vi "RANGE Gas Meters.vi"() -> ()   [LabVIEW 2023]
uses:
  Type Definitions/RANGE DAQ Data Four Meters.ctl
  Type Definitions/RANGE DAQ Data.ctl
  Drivers/Omega FMA-1600A Series Gas Flow Meter/Type Definitions/FMA1600A Gas Type.ctl
  Drivers/Omega FMA-1600A Series Gas Flow Meter/Type Definitions/FMA1600A Units String.ctl
  Drivers/Alicat Gas Meter Driver/Sub-VIs/Units of Measure.ctl
  Drivers/Alicat Gas Meter Driver/Sub-VIs/Data Frame.ctl
  Type Definitions/RANGE GAS Data.ctl
  Type Definitions/RANGE Panel Data.ctl
  Type Definitions/RANGE ANSI Rate.ctl
  Type Definitions/RANGE Meter Selector 1-2.ctl
  Type Definitions/RANGE Meter Selector 3-4.ctl
  Type Definitions/RANGE Meter Selector 5-6.ctl
  Type Definitions/RANGE Tab Control 2.ctl
  Drivers/Omega FMA-1600A Series Gas Flow Meter/Type Definitions/FMA1600A Commands.ctl
  ValveTester/LabVIEW/Controls/GLVT-Stepper-EnableState.ctl
  ValveTester/LabVIEW/Controls/GLVT-FlowmeterBankSelection.ctl
  ValveTester/LabVIEW/Controls/GLVT-Stepper-RotateDirection.ctl
  Drivers/Inficon Fusion Micro GC/Type Definitions/Inficon IP Address.ctl
  <vilib>/NI/Modbus Library/API/Master/Modbus Master.lvclass
  Utility/Type Definitions/UTILITY Notifier.ctl
  ValveTester/LabVIEW/Controls/GLVT-States.ctl
  Utility/Custom Pallet Controls/Custom Pallet DBL.ctl
  ValveTester/LabVIEW/Controls/GLVT-FGV-States.ctl
  Type Definitions/Range Meter Bank.ctl
  <vilib>/Analysis/baseanly.llb/Mean (DBL).vi
  <vilib>/Analysis/NI_AALBase.lvlib
panel:
  out "GLVT-Filename DTS":string caption="Filename DTS"
  out "GLVT-End Data Collection":bool caption="End Data Collection"
  out "GLVT-Current Angle Array Location":i32 caption="Current Angle Array Location"
  out "GLVT-Row Length":i32
  out "GLVT-Rotate Direction":T1 caption="Rotate Direction"
  in  "Tab Control 2":T2
  out "Bank 3 Gas Pres 2":string
  out "Bank 3 Gas Temp 2":string
  out "Bank 3 Tot. Flow 2":string
  out "Bank 3 Vol Flow 2":string
  out "Bank 3 Mass Flow 2":string
  out "Bank 2 Gas Pres":string
  out "Bank 2 Gas Temp":string
  out "Bank 2 Tot. Flow":string
  out "Bank 2 Vol Flow":string
  out "Bank 2 Mass Flow":string
  out "Bank 1 Gas Pres 2":string
  out "Bank 1 Gas Temp 2":string
  out "Bank 1 Tot. Flow 2":string
  out "Bank 1 Vol Flow 2":string
  in  "Tare Meter Bank 3":bool
  in  "Reset Totalizer Bank 3":bool
  in  "Change Gas Meter Bank 3":bool
  in  "Gas Type 3":T3
  in  "Tare Meter Bank 2":bool
  in  "Reset Totalizer Bank 2":bool
  in  "Change Gas Meter Bank 2":bool
  in  "Gas Type 2":T3
  in  "Tare Meter Bank 1":bool
  in  "Reset Totalizer Bank 1":bool
  out "Flow Rate":dbl caption="Flow Rate (BTU/hr)" format="%#_5f"
  out "DisplayChart":cluster{"Flow Rate (BTU/HR)":dbl}(graph)
  in  "HeatingValueS1":dbl=2450.0 min=2400.0 max=2600.0 step=1.0
  in  "Meter Select":T4
  out "Flow Rate 2":dbl caption="Flow Rate (BTU/hr)" format="%#_5f"
  out "DisplayChart 2":cluster{"Flow Rate (BTU/HR)":dbl}(graph)
  in  "HeatingValueS2":dbl=2450.0 min=900.0 max=2600.0 step=1.0
  in  "Meter Select 2":T5 caption="Meter Select"
  out "Flow Rate 3":dbl caption="Flow Rate (BTU/hr)" format="%#_5f"
  out "DisplayChart 3":cluster{"Flow Rate (BTU/HR)":dbl}(graph)
  in  "HeatingValueS3":dbl=2450.0 min=900.0 max=2600.0 step=1.0
  in  "Meter Select 3":T6 caption="Meter Select"
  out "Display Bank 2":T7
  out "Display Bank 3":T7
  out "ANSI Display 3":string
  in  "Start ANSI 3":bool
  out "ANSI Average (BTU/hr) 3":dbl caption="ANSI Average (BTU/hr)" format="%#_5g"
  out "ANSI Display 2":string
  in  "Start ANSI 2":bool
  out "ANSI Average (BTU/hr) 2":dbl caption="ANSI Average (BTU/hr)" format="%#_5g"
  out "ANSI Display 1":string
  in  "Start ANSI":bool
  out "ANSI Average (BTU/hr)":dbl format="%#_5g"
  in  "Change Gas Meter Bank1":bool
  in  "Gas Type":T3
  out "Bank 1 Mass Flow 2":string
  out "Display Bank 1":T7
  out "Meter Software 1/2":string
  out "Meter Software 3/4":string
  out "Meter Software 5/6":string
  in  "Manual HHV 1":bool=TRUE caption="Manual HHV"
  in  "Manual HHV 2":bool=TRUE caption="Manual HHV"
  in  "Manual HHV 3":bool=TRUE caption="Manual HHV"
  out "Bank 1 Tot. Flow":string
  out "Bank 1 Gas Pres":string
  out "Bank 1 Gas Temp":string
  out "Bank 1 Vol Flow":string
  out "Bank 1 Mass Flow":string
  out "Display S1":T8
  out "Station 1 Chart":cluster{"Flow Rate (BTU/HR)":dbl}(graph)
  out "Flow Rate S1":dbl caption="Flow Rate (BTU/hr)" format="%#_5g"
  out "ANSI Display S1":string caption="ANSI Display 1"
  in  "Start ANSI-S1":bool
  out "ANSI Average (BTU/hr)-Meter 1/2":dbl format="%#_5g"
  in  "HeatingValue Meter 1/2":dbl=2450.0 min=2400.0 max=2600.0 step=1.0
  in  "Meter Select 1/2":T4
  out "Meter 1/2":string caption="Meter"
  out "Bank 2 Mass Flow 2":string
  out "Bank 2 Vol Flow 3":string
  out "Bank 2 Gas Temp 3":string
  out "Bank 2 Gas Pres 3":string
  out "Bank 2 Tot. Flow 3":string
  out "Station 2 Chart":cluster{"Flow Rate (BTU/HR)":dbl}(graph)
  out "ANSI Display S2":string caption="ANSI Display 1"
  in  "Start ANSI-S2":bool
  out "ANSI Average (BTU/hr)-Meter 3/4":dbl format="%#_5g"
  out "Flow Rate S2":dbl caption="Flow Rate (BTU/hr)" format="%#_5g"
  out "Display S2":T8
  in  "HeatingValue Meter 3/4":dbl=2450.0 min=2400.0 max=2600.0 step=1.0
  in  "Meter Select 3/4":T5 caption="Meter Select 3-4"
  out "Meter 3/4":string caption="Meter"
  out "Bank 3 Mass Flow":string
  out "Bank 3 Vol Flow":string
  out "Bank 3 Gas Temp":string
  out "Bank 3 Gas Pres":string
  out "Bank 3 Tot. Flow":string
  out "Station 3 Chart":cluster{"Flow Rate (BTU/HR)":dbl}(graph)
  out "Flow Rate S3":dbl caption="Flow Rate (BTU/hr)" format="%#_5g"
  out "ANSI Display S3":string caption="ANSI Display 1"
  in  "Start ANSI-S3":bool
  out "ANSI Average (BTU/hr)-Meter 5/6":dbl format="%#_5g"
  out "Display S3":T8
  in  "HeatingValue Meter 5/6":dbl=2450.0 min=2400.0 max=2600.0 step=1.0
  in  "Meter Select 5/6":T6 caption="Meter Select 5-6"
  out "Meter 5/6":string caption="Meter"
  in  "Manual Commands":bool
  in  "Tab Control 3":T9(tab)
  in  "FMA1600A Commands":T10="*w42=31730"
  out "Raw FMA1600A Data":string
  in  "Unit ID (A-F)":string
  out "GLVT-Angle for Gas Stop":dbl caption="Angle for Gas Stop"
  out "GLVT-Angle for Gas Start":dbl caption="Angle for Gas Start"
  out "GLVT-Working":bool caption="Working"
  out "GLVT-Angles for Data Collection (deg abs)":dbl[](array[numeric]) caption="Angles for Data Collection (deg abs)"
  in  "GLVT-Measure Valve Button":bool caption="Measure Valve Button"
  in  "GLVT-Angle per Step":dbl=1.0 caption="Angle per Step" min=1.0 max=360.0 step=0.1
  in  "GLVT-Max Angle to Rotate (deg abs)":dbl caption="Max Angle to Rotate (deg abs)" min=0.0 max=360.0 step=0.1
  in  "GLVT-Data Measure Time":dbl=1.0 caption="Data Measure Time" min=1.0 step=0.1 format="%<%H:%M:%S>t"
  out "GLVT-Motor Position Actual":dbl caption="Motor Position Actual" format="%#.2f"
  in  "GLVT-Move Stepper Button":bool caption="Move Stepper Button"
  in  "GLVT-Angle to Rotate  (deg abs)":dbl caption="Angle to Rotate  (deg abs)" step=0.1
  in  "GLVT-Motor State":T11 caption="Motor State"
  in  "GLVT-Release Motor Button":bool
  in  "GLVT-Pulse Rate (pps)":i32=600 caption="Pulse Rate (pps)"
  in  "GLVT-Steps per Rev":i32=1600 caption="Steps per Rev"
  in  "GLVT-Flowmeter Bank":T12 caption="Flowmeter Bank"
  out "GLVT-Collected Data":cluster{"Data Out":dbl[], "Data Out":dbl[]}[](graph) caption="Collected Data"
  out "GLVT-Save Data Location":path caption="Save Data Location"
  in  "GLVT-Filename Descriptor":string caption="Filename Descriptor"
  in  "Scan Rate (Sec)":dbl=1.0
  in  "Exit Button":bool
  out "Elapsed Time":dbl format="%<%H:%M:%S>t"
  out "File  Version":string="Parametric Stand"
  in  "Record":bool
  in  "File Path":path
  in  "Tab Control":enum32{"Debug Data", "Page 2", "Page 3"}(tab)
  out "Error Out":errorcluster
  in  "Error In":errorcluster
  out "All Meter Data":T13={"Meter 1"={"Meter Size"=0.0, "DAQ Output (Voltage)"=0.0, "Reference (Voltage)"=0.0, "Meter Present"=FALSE, "Meter Visa"="COM3", "Gas Type"="12", "SLPM Error @ Zero"=0.0, "Gas Mix Number"="", "Set STP Register"=FALSE, "Measurement Units"={"Software Rev"="", "Model Number"="", "Manufacturer Info"="", "Software Sub-Rev"="", "Board Rev"="", "Units of Measure Input"={"Abs. Pressure"="", "Gauge/Diff. Press."="", "Barometric Press."="", "Temperature"="", "Volume"="", "Mass"="", "Setpoint"="", "Valve Drive"="", "Totalizer"="", "Tot. Timer"="", "Tot. Avg. Flow"="", "Tot. Peak Flow"=""}}, "Data Frame Format"={"Absolute Pressure"=FALSE, "Gauge/Diff. Pressure"=FALSE, "Barometric Pressure"=FALSE, "Temperature"=FALSE, "Volumetric"=FALSE, "Mass"=FALSE, "Setpoint"=FALSE, "Valve Drive"=FALSE, "Totalizer"=FALSE, "Totalizer Timer"=FALSE, "Totalizer Average Flow"=FALSE, "Totalizer Peak Flow"=FALSE, "Gas Selected"=FALSE, "Tot. Timer Format"=0}}, "Meter 2"={"Meter Size"=0.0, "DAQ Output (Voltage)"=0.0, "Reference (Voltage)"=0.0, "Meter Present"=FALSE, "Meter Visa"="COM3", "Gas Type"="12", "SLPM Error @ Zero"=0.0, "Gas Mix Number"="", "Set STP Register"=FALSE, "Measurement Units"={"Software Rev"="", "Model Number"="", "Manufacturer Info"="", "Software Sub-Rev"="", "Board Rev"="", "Units of Measure Input"={"Abs. Pressure"="", "Gauge/Diff. Press."="", "Barometric Press."="", "Temperature"="", "Volume"="", "Mass"="", "Setpoint"="", "Valve Drive"="", "Totalizer"="", "Tot. Timer"="", "Tot. Avg. Flow"="", "Tot. Peak Flow"=""}}, "Data Frame Format"={"Absolute Pressure"=FALSE, "Gauge/Diff. Pressure"=FALSE, "Barometric Pressure"=FALSE, "Temperature"=FALSE, "Volumetric"=FALSE, "Mass"=FALSE, "Setpoint"=FALSE, "Valve Drive"=FALSE, "Totalizer"=FALSE, "Totalizer Timer"=FALSE, "Totalizer Average Flow"=FALSE, "Totalizer Peak Flow"=FALSE, "Gas Selected"=FALSE, "Tot. Timer Format"=0}}, "Meter 3"={"Meter Size"=0.0, "DAQ Output (Voltage)"=0.0, "Reference (Voltage)"=0.0, "Meter Present"=FALSE, "Meter Visa"="COM3", "Gas Type"="12", "SLPM Error @ Zero"=0.0, "Gas Mix Number"="", "Set STP Register"=FALSE, "Measurement Units"={"Software Rev"="", "Model Number"="", "Manufacturer Info"="", "Software Sub-Rev"="", "Board Rev"="", "Units of Measure Input"={"Abs. Pressure"="", "Gauge/Diff. Press."="", "Barometric Press."="", "Temperature"="", "Volume"="", "Mass"="", "Setpoint"="", "Valve Drive"="", "Totalizer"="", "Tot. Timer"="", "Tot. Avg. Flow"="", "Tot. Peak Flow"=""}}, "Data Frame Format"={"Absolute Pressure"=FALSE, "Gauge/Diff. Pressure"=FALSE, "Barometric Pressure"=FALSE, "Temperature"=FALSE, "Volumetric"=FALSE, "Mass"=FALSE, "Setpoint"=FALSE, "Valve Drive"=FALSE, "Totalizer"=FALSE, "Totalizer Timer"=FALSE, "Totalizer Average Flow"=FALSE, "Totalizer Peak Flow"=FALSE, "Gas Selected"=FALSE, "Tot. Timer Format"=0}}, "Meter 4"={"Meter Size"=0.0, "DAQ Output (Voltage)"=0.0, "Reference (Voltage)"=0.0, "Meter Present"=FALSE, "Meter Visa"="COM3", "Gas Type"="12", "SLPM Error @ Zero"=0.0, "Gas Mix Number"="", "Set STP Register"=FALSE, "Measurement Units"={"Software Rev"="", "Model Number"="", "Manufacturer Info"="", "Software Sub-Rev"="", "Board Rev"="", "Units of Measure Input"={"Abs. Pressure"="", "Gauge/Diff. Press."="", "Barometric Press."="", "Temperature"="", "Volume"="", "Mass"="", "Setpoint"="", "Valve Drive"="", "Totalizer"="", "Tot. Timer"="", "Tot. Avg. Flow"="", "Tot. Peak Flow"=""}}, "Data Frame Format"={"Absolute Pressure"=FALSE, "Gauge/Diff. Pressure"=FALSE, "Barometric Pressure"=FALSE, "Temperature"=FALSE, "Volumetric"=FALSE, "Mass"=FALSE, "Setpoint"=FALSE, "Valve Drive"=FALSE, "Totalizer"=FALSE, "Totalizer Timer"=FALSE, "Totalizer Average Flow"=FALSE, "Totalizer Peak Flow"=FALSE, "Gas Selected"=FALSE, "Tot. Timer Format"=0}}, "Meter 5"={"Meter Size"=0.0, "DAQ Output (Voltage)"=0.0, "Reference (Voltage)"=0.0, "Meter Present"=FALSE, "Meter Visa"="COM3", "Gas Type"="12", "SLPM Error @ Zero"=0.0, "Gas Mix Number"="", "Set STP Register"=FALSE, "Measurement Units"={"Software Rev"="", "Model Number"="", "Manufacturer Info"="", "Software Sub-Rev"="", "Board Rev"="", "Units of Measure Input"={"Abs. Pressure"="", "Gauge/Diff. Press."="", "Barometric Press."="", "Temperature"="", "Volume"="", "Mass"="", "Setpoint"="", "Valve Drive"="", "Totalizer"="", "Tot. Timer"="", "Tot. Avg. Flow"="", "Tot. Peak Flow"=""}}, "Data Frame Format"={"Absolute Pressure"=FALSE, "Gauge/Diff. Pressure"=FALSE, "Barometric Pressure"=FALSE, "Temperature"=FALSE, "Volumetric"=FALSE, "Mass"=FALSE, "Setpoint"=FALSE, "Valve Drive"=FALSE, "Totalizer"=FALSE, "Totalizer Timer"=FALSE, "Totalizer Average Flow"=FALSE, "Totalizer Peak Flow"=FALSE, "Gas Selected"=FALSE, "Tot. Timer Format"=0}}, "Meter 6"={"Meter Size"=0.0, "DAQ Output (Voltage)"=0.0, "Reference (Voltage)"=0.0, "Meter Present"=FALSE, "Meter Visa"="COM3", "Gas Type"="12", "SLPM Error @ Zero"=0.0, "Gas Mix Number"="", "Set STP Register"=FALSE, "Measurement Units"={"Software Rev"="", "Model Number"="", "Manufacturer Info"="", "Software Sub-Rev"="", "Board Rev"="", "Units of Measure Input"={"Abs. Pressure"="", "Gauge/Diff. Press."="", "Barometric Press."="", "Temperature"="", "Volume"="", "Mass"="", "Setpoint"="", "Valve Drive"="", "Totalizer"="", "Tot. Timer"="", "Tot. Avg. Flow"="", "Tot. Peak Flow"=""}}, "Data Frame Format"={"Absolute Pressure"=FALSE, "Gauge/Diff. Pressure"=FALSE, "Barometric Pressure"=FALSE, "Temperature"=FALSE, "Volumetric"=FALSE, "Mass"=FALSE, "Setpoint"=FALSE, "Valve Drive"=FALSE, "Totalizer"=FALSE, "Totalizer Timer"=FALSE, "Totalizer Average Flow"=FALSE, "Totalizer Peak Flow"=FALSE, "Gas Selected"=FALSE, "Tot. Timer Format"=0}}, "Meter Bank 1"={"Flow Rate (BTU/HR)"=0.0, "ANSI Average (BTU/HR)"=0.0, "Panel Data"={"Meter Type (Gas)"="", "Heating Value (BTU/ft³)"=0.0, "Ft³ / Hr (SCFH)"=0.0, "15 Second Average (BTU/HR)"=0.0, "30 Second Average (BTU/HR)"=0.0, "Mass Flow"=0.0, "Vol. Flow"=0.0, "Gas Temperature"=0.0, "Gas Pressure"=0.0, "Tot.Flow"=0.0}, "Meter ID"="", "ANSI Rate"={"Array 1"=[], "Array 3"=[], "Array 2"=[], "Start ANSI"=FALSE, "ANSI Start Time"=0.0, "Restart ANSI"=FALSE, "15 Min ANSI Avg (BTU/hr)"=0.0, "20 Min ANSI Avg (BTU/hr)"=0.0, "25 Min ANSI Avg (BTU/hr)"=0.0, "Absolute Pressure"=0.0, "Gas Temperature"=0.0, "Volumetric Flow Rate"=0.0, "Mass Flow Rate"=0.0, "Array 4"=[], "Array 5"=[], "Gas Rate"=0.0, "15 Min Pres Avg (PSIA)"=0.0, "20 Min Pres Avg (PSIA)"=0.0, "25 Min Pres Avg (PSIA)"=0.0, "15 Min Temp Avg (°F) "=0.0, "20 Min Temp Avg (°F)"=0.0, "25 Min Temp Avg (°F)"=0.0, "15 Min Uncorrected Avg (CFH)"=0.0, "20 Min Uncorrected Avg (CFH)"=0.0, "25 Min Uncorrected Avg (CFH)"=0.0, "15 Min Corrected Avg (SCFH)"=0.0, "20 Min Corrected Avg (SCFH)"=0.0, "25 Min Corrected Avg (SCFH)"=0.0, "15 Min Complete"=FALSE, "20 Min Complete"=FALSE, "25 Min Complete"=FALSE, "Heating Value (BTU/ft³)"=0.0, "CO CO2 15 Min"=[], "CO CO2 20 Min"=[], "CO CO2 25 Min"=[], "CO CO2 Real Time"=[]}}, "Meter Bank 2"={"Flow Rate (BTU/HR)"=0.0, "ANSI Average (BTU/HR)"=0.0, "Panel Data"={"Meter Type (Gas)"="", "Heating Value (BTU/ft³)"=0.0, "Ft³ / Hr (SCFH)"=0.0, "15 Second Average (BTU/HR)"=0.0, "30 Second Average (BTU/HR)"=0.0, "Mass Flow"=0.0, "Vol. Flow"=0.0, "Gas Temperature"=0.0, "Gas Pressure"=0.0, "Tot.Flow"=0.0}, "Meter ID"="", "ANSI Rate"={"Array 1"=[], "Array 3"=[], "Array 2"=[], "Start ANSI"=FALSE, "ANSI Start Time"=0.0, "Restart ANSI"=FALSE, "15 Min ANSI Avg (BTU/hr)"=0.0, "20 Min ANSI Avg (BTU/hr)"=0.0, "25 Min ANSI Avg (BTU/hr)"=0.0, "Absolute Pressure"=0.0, "Gas Temperature"=0.0, "Volumetric Flow Rate"=0.0, "Mass Flow Rate"=0.0, "Array 4"=[], "Array 5"=[], "Gas Rate"=0.0, "15 Min Pres Avg (PSIA)"=0.0, "20 Min Pres Avg (PSIA)"=0.0, "25 Min Pres Avg (PSIA)"=0.0, "15 Min Temp Avg (°F) "=0.0, "20 Min Temp Avg (°F)"=0.0, "25 Min Temp Avg (°F)"=0.0, "15 Min Uncorrected Avg (CFH)"=0.0, "20 Min Uncorrected Avg (CFH)"=0.0, "25 Min Uncorrected Avg (CFH)"=0.0, "15 Min Corrected Avg (SCFH)"=0.0, "20 Min Corrected Avg (SCFH)"=0.0, "25 Min Corrected Avg (SCFH)"=0.0, "15 Min Complete"=FALSE, "20 Min Complete"=FALSE, "25 Min Complete"=FALSE, "Heating Value (BTU/ft³)"=0.0, "CO CO2 15 Min"=[], "CO CO2 20 Min"=[], "CO CO2 25 Min"=[], "CO CO2 Real Time"=[]}}, "Meter Bank 3"={"Flow Rate (BTU/HR)"=0.0, "ANSI Average (BTU/HR)"=0.0, "Panel Data"={"Meter Type (Gas)"="", "Heating Value (BTU/ft³)"=0.0, "Ft³ / Hr (SCFH)"=0.0, "15 Second Average (BTU/HR)"=0.0, "30 Second Average (BTU/HR)"=0.0, "Mass Flow"=0.0, "Vol. Flow"=0.0, "Gas Temperature"=0.0, "Gas Pressure"=0.0, "Tot.Flow"=0.0}, "Meter ID"="", "ANSI Rate"={"Array 1"=[], "Array 3"=[], "Array 2"=[], "Start ANSI"=FALSE, "ANSI Start Time"=0.0, "Restart ANSI"=FALSE, "15 Min ANSI Avg (BTU/hr)"=0.0, "20 Min ANSI Avg (BTU/hr)"=0.0, "25 Min ANSI Avg (BTU/hr)"=0.0, "Absolute Pressure"=0.0, "Gas Temperature"=0.0, "Volumetric Flow Rate"=0.0, "Mass Flow Rate"=0.0, "Array 4"=[], "Array 5"=[], "Gas Rate"=0.0, "15 Min Pres Avg (PSIA)"=0.0, "20 Min Pres Avg (PSIA)"=0.0, "25 Min Pres Avg (PSIA)"=0.0, "15 Min Temp Avg (°F) "=0.0, "20 Min Temp Avg (°F)"=0.0, "25 Min Temp Avg (°F)"=0.0, "15 Min Uncorrected Avg (CFH)"=0.0, "20 Min Uncorrected Avg (CFH)"=0.0, "25 Min Uncorrected Avg (CFH)"=0.0, "15 Min Corrected Avg (SCFH)"=0.0, "20 Min Corrected Avg (SCFH)"=0.0, "25 Min Corrected Avg (SCFH)"=0.0, "15 Min Complete"=FALSE, "20 Min Complete"=FALSE, "25 Min Complete"=FALSE, "Heating Value (BTU/ft³)"=0.0, "CO CO2 15 Min"=[], "CO CO2 20 Min"=[], "CO CO2 25 Min"=[], "CO CO2 Real Time"=[]}}, "Threshold Voltage (NI DAQ)"=0.2, "Use RS232 Data Collection"=FALSE, "Use Auto Switching"=FALSE}
  out "Main Loop Rate":dbl format="%0.2f"
  out "Tot.Flow (SLPM Liters) Bank 1":dbl
  out "Tot.Flow (SLPM Liters) Bank 2":dbl
  out "Tot.Flow (SLPM Liters) Bank 3":dbl
  out "Average Updates":T13={"Meter 1"={"Meter Size"=0.0, "DAQ Output (Voltage)"=0.0, "Reference (Voltage)"=0.0, "Meter Present"=FALSE, "Meter Visa"="COM3", "Gas Type"="12", "SLPM Error @ Zero"=0.0, "Gas Mix Number"="", "Set STP Register"=FALSE, "Measurement Units"={"Software Rev"="", "Model Number"="", "Manufacturer Info"="", "Software Sub-Rev"="", "Board Rev"="", "Units of Measure Input"={"Abs. Pressure"="", "Gauge/Diff. Press."="", "Barometric Press."="", "Temperature"="", "Volume"="", "Mass"="", "Setpoint"="", "Valve Drive"="", "Totalizer"="", "Tot. Timer"="", "Tot. Avg. Flow"="", "Tot. Peak Flow"=""}}, "Data Frame Format"={"Absolute Pressure"=FALSE, "Gauge/Diff. Pressure"=FALSE, "Barometric Pressure"=FALSE, "Temperature"=FALSE, "Volumetric"=FALSE, "Mass"=FALSE, "Setpoint"=FALSE, "Valve Drive"=FALSE, "Totalizer"=FALSE, "Totalizer Timer"=FALSE, "Totalizer Average Flow"=FALSE, "Totalizer Peak Flow"=FALSE, "Gas Selected"=FALSE, "Tot. Timer Format"=0}}, "Meter 2"={"Meter Size"=0.0, "DAQ Output (Voltage)"=0.0, "Reference (Voltage)"=0.0, "Meter Present"=FALSE, "Meter Visa"="COM3", "Gas Type"="12", "SLPM Error @ Zero"=0.0, "Gas Mix Number"="", "Set STP Register"=FALSE, "Measurement Units"={"Software Rev"="", "Model Number"="", "Manufacturer Info"="", "Software Sub-Rev"="", "Board Rev"="", "Units of Measure Input"={"Abs. Pressure"="", "Gauge/Diff. Press."="", "Barometric Press."="", "Temperature"="", "Volume"="", "Mass"="", "Setpoint"="", "Valve Drive"="", "Totalizer"="", "Tot. Timer"="", "Tot. Avg. Flow"="", "Tot. Peak Flow"=""}}, "Data Frame Format"={"Absolute Pressure"=FALSE, "Gauge/Diff. Pressure"=FALSE, "Barometric Pressure"=FALSE, "Temperature"=FALSE, "Volumetric"=FALSE, "Mass"=FALSE, "Setpoint"=FALSE, "Valve Drive"=FALSE, "Totalizer"=FALSE, "Totalizer Timer"=FALSE, "Totalizer Average Flow"=FALSE, "Totalizer Peak Flow"=FALSE, "Gas Selected"=FALSE, "Tot. Timer Format"=0}}, "Meter 3"={"Meter Size"=0.0, "DAQ Output (Voltage)"=0.0, "Reference (Voltage)"=0.0, "Meter Present"=FALSE, "Meter Visa"="COM3", "Gas Type"="12", "SLPM Error @ Zero"=0.0, "Gas Mix Number"="", "Set STP Register"=FALSE, "Measurement Units"={"Software Rev"="", "Model Number"="", "Manufacturer Info"="", "Software Sub-Rev"="", "Board Rev"="", "Units of Measure Input"={"Abs. Pressure"="", "Gauge/Diff. Press."="", "Barometric Press."="", "Temperature"="", "Volume"="", "Mass"="", "Setpoint"="", "Valve Drive"="", "Totalizer"="", "Tot. Timer"="", "Tot. Avg. Flow"="", "Tot. Peak Flow"=""}}, "Data Frame Format"={"Absolute Pressure"=FALSE, "Gauge/Diff. Pressure"=FALSE, "Barometric Pressure"=FALSE, "Temperature"=FALSE, "Volumetric"=FALSE, "Mass"=FALSE, "Setpoint"=FALSE, "Valve Drive"=FALSE, "Totalizer"=FALSE, "Totalizer Timer"=FALSE, "Totalizer Average Flow"=FALSE, "Totalizer Peak Flow"=FALSE, "Gas Selected"=FALSE, "Tot. Timer Format"=0}}, "Meter 4"={"Meter Size"=0.0, "DAQ Output (Voltage)"=0.0, "Reference (Voltage)"=0.0, "Meter Present"=FALSE, "Meter Visa"="COM3", "Gas Type"="12", "SLPM Error @ Zero"=0.0, "Gas Mix Number"="", "Set STP Register"=FALSE, "Measurement Units"={"Software Rev"="", "Model Number"="", "Manufacturer Info"="", "Software Sub-Rev"="", "Board Rev"="", "Units of Measure Input"={"Abs. Pressure"="", "Gauge/Diff. Press."="", "Barometric Press."="", "Temperature"="", "Volume"="", "Mass"="", "Setpoint"="", "Valve Drive"="", "Totalizer"="", "Tot. Timer"="", "Tot. Avg. Flow"="", "Tot. Peak Flow"=""}}, "Data Frame Format"={"Absolute Pressure"=FALSE, "Gauge/Diff. Pressure"=FALSE, "Barometric Pressure"=FALSE, "Temperature"=FALSE, "Volumetric"=FALSE, "Mass"=FALSE, "Setpoint"=FALSE, "Valve Drive"=FALSE, "Totalizer"=FALSE, "Totalizer Timer"=FALSE, "Totalizer Average Flow"=FALSE, "Totalizer Peak Flow"=FALSE, "Gas Selected"=FALSE, "Tot. Timer Format"=0}}, "Meter 5"={"Meter Size"=0.0, "DAQ Output (Voltage)"=0.0, "Reference (Voltage)"=0.0, "Meter Present"=FALSE, "Meter Visa"="COM3", "Gas Type"="12", "SLPM Error @ Zero"=0.0, "Gas Mix Number"="", "Set STP Register"=FALSE, "Measurement Units"={"Software Rev"="", "Model Number"="", "Manufacturer Info"="", "Software Sub-Rev"="", "Board Rev"="", "Units of Measure Input"={"Abs. Pressure"="", "Gauge/Diff. Press."="", "Barometric Press."="", "Temperature"="", "Volume"="", "Mass"="", "Setpoint"="", "Valve Drive"="", "Totalizer"="", "Tot. Timer"="", "Tot. Avg. Flow"="", "Tot. Peak Flow"=""}}, "Data Frame Format"={"Absolute Pressure"=FALSE, "Gauge/Diff. Pressure"=FALSE, "Barometric Pressure"=FALSE, "Temperature"=FALSE, "Volumetric"=FALSE, "Mass"=FALSE, "Setpoint"=FALSE, "Valve Drive"=FALSE, "Totalizer"=FALSE, "Totalizer Timer"=FALSE, "Totalizer Average Flow"=FALSE, "Totalizer Peak Flow"=FALSE, "Gas Selected"=FALSE, "Tot. Timer Format"=0}}, "Meter 6"={"Meter Size"=0.0, "DAQ Output (Voltage)"=0.0, "Reference (Voltage)"=0.0, "Meter Present"=FALSE, "Meter Visa"="COM3", "Gas Type"="12", "SLPM Error @ Zero"=0.0, "Gas Mix Number"="", "Set STP Register"=FALSE, "Measurement Units"={"Software Rev"="", "Model Number"="", "Manufacturer Info"="", "Software Sub-Rev"="", "Board Rev"="", "Units of Measure Input"={"Abs. Pressure"="", "Gauge/Diff. Press."="", "Barometric Press."="", "Temperature"="", "Volume"="", "Mass"="", "Setpoint"="", "Valve Drive"="", "Totalizer"="", "Tot. Timer"="", "Tot. Avg. Flow"="", "Tot. Peak Flow"=""}}, "Data Frame Format"={"Absolute Pressure"=FALSE, "Gauge/Diff. Pressure"=FALSE, "Barometric Pressure"=FALSE, "Temperature"=FALSE, "Volumetric"=FALSE, "Mass"=FALSE, "Setpoint"=FALSE, "Valve Drive"=FALSE, "Totalizer"=FALSE, "Totalizer Timer"=FALSE, "Totalizer Average Flow"=FALSE, "Totalizer Peak Flow"=FALSE, "Gas Selected"=FALSE, "Tot. Timer Format"=0}}, "Meter Bank 1"={"Flow Rate (BTU/HR)"=0.0, "ANSI Average (BTU/HR)"=0.0, "Panel Data"={"Meter Type (Gas)"="", "Heating Value (BTU/ft³)"=0.0, "Ft³ / Hr (SCFH)"=0.0, "15 Second Average (BTU/HR)"=0.0, "30 Second Average (BTU/HR)"=0.0, "Mass Flow"=0.0, "Vol. Flow"=0.0, "Gas Temperature"=0.0, "Gas Pressure"=0.0, "Tot.Flow"=0.0}, "Meter ID"="", "ANSI Rate"={"Array 1"=[], "Array 3"=[], "Array 2"=[], "Start ANSI"=FALSE, "ANSI Start Time"=0.0, "Restart ANSI"=FALSE, "15 Min ANSI Avg (BTU/hr)"=0.0, "20 Min ANSI Avg (BTU/hr)"=0.0, "25 Min ANSI Avg (BTU/hr)"=0.0, "Absolute Pressure"=0.0, "Gas Temperature"=0.0, "Volumetric Flow Rate"=0.0, "Mass Flow Rate"=0.0, "Array 4"=[], "Array 5"=[], "Gas Rate"=0.0, "15 Min Pres Avg (PSIA)"=0.0, "20 Min Pres Avg (PSIA)"=0.0, "25 Min Pres Avg (PSIA)"=0.0, "15 Min Temp Avg (°F) "=0.0, "20 Min Temp Avg (°F)"=0.0, "25 Min Temp Avg (°F)"=0.0, "15 Min Uncorrected Avg (CFH)"=0.0, "20 Min Uncorrected Avg (CFH)"=0.0, "25 Min Uncorrected Avg (CFH)"=0.0, "15 Min Corrected Avg (SCFH)"=0.0, "20 Min Corrected Avg (SCFH)"=0.0, "25 Min Corrected Avg (SCFH)"=0.0, "15 Min Complete"=FALSE, "20 Min Complete"=FALSE, "25 Min Complete"=FALSE, "Heating Value (BTU/ft³)"=0.0, "CO CO2 15 Min"=[], "CO CO2 20 Min"=[], "CO CO2 25 Min"=[], "CO CO2 Real Time"=[]}}, "Meter Bank 2"={"Flow Rate (BTU/HR)"=0.0, "ANSI Average (BTU/HR)"=0.0, "Panel Data"={"Meter Type (Gas)"="", "Heating Value (BTU/ft³)"=0.0, "Ft³ / Hr (SCFH)"=0.0, "15 Second Average (BTU/HR)"=0.0, "30 Second Average (BTU/HR)"=0.0, "Mass Flow"=0.0, "Vol. Flow"=0.0, "Gas Temperature"=0.0, "Gas Pressure"=0.0, "Tot.Flow"=0.0}, "Meter ID"="", "ANSI Rate"={"Array 1"=[], "Array 3"=[], "Array 2"=[], "Start ANSI"=FALSE, "ANSI Start Time"=0.0, "Restart ANSI"=FALSE, "15 Min ANSI Avg (BTU/hr)"=0.0, "20 Min ANSI Avg (BTU/hr)"=0.0, "25 Min ANSI Avg (BTU/hr)"=0.0, "Absolute Pressure"=0.0, "Gas Temperature"=0.0, "Volumetric Flow Rate"=0.0, "Mass Flow Rate"=0.0, "Array 4"=[], "Array 5"=[], "Gas Rate"=0.0, "15 Min Pres Avg (PSIA)"=0.0, "20 Min Pres Avg (PSIA)"=0.0, "25 Min Pres Avg (PSIA)"=0.0, "15 Min Temp Avg (°F) "=0.0, "20 Min Temp Avg (°F)"=0.0, "25 Min Temp Avg (°F)"=0.0, "15 Min Uncorrected Avg (CFH)"=0.0, "20 Min Uncorrected Avg (CFH)"=0.0, "25 Min Uncorrected Avg (CFH)"=0.0, "15 Min Corrected Avg (SCFH)"=0.0, "20 Min Corrected Avg (SCFH)"=0.0, "25 Min Corrected Avg (SCFH)"=0.0, "15 Min Complete"=FALSE, "20 Min Complete"=FALSE, "25 Min Complete"=FALSE, "Heating Value (BTU/ft³)"=0.0, "CO CO2 15 Min"=[], "CO CO2 20 Min"=[], "CO CO2 25 Min"=[], "CO CO2 Real Time"=[]}}, "Meter Bank 3"={"Flow Rate (BTU/HR)"=0.0, "ANSI Average (BTU/HR)"=0.0, "Panel Data"={"Meter Type (Gas)"="", "Heating Value (BTU/ft³)"=0.0, "Ft³ / Hr (SCFH)"=0.0, "15 Second Average (BTU/HR)"=0.0, "30 Second Average (BTU/HR)"=0.0, "Mass Flow"=0.0, "Vol. Flow"=0.0, "Gas Temperature"=0.0, "Gas Pressure"=0.0, "Tot.Flow"=0.0}, "Meter ID"="", "ANSI Rate"={"Array 1"=[], "Array 3"=[], "Array 2"=[], "Start ANSI"=FALSE, "ANSI Start Time"=0.0, "Restart ANSI"=FALSE, "15 Min ANSI Avg (BTU/hr)"=0.0, "20 Min ANSI Avg (BTU/hr)"=0.0, "25 Min ANSI Avg (BTU/hr)"=0.0, "Absolute Pressure"=0.0, "Gas Temperature"=0.0, "Volumetric Flow Rate"=0.0, "Mass Flow Rate"=0.0, "Array 4"=[], "Array 5"=[], "Gas Rate"=0.0, "15 Min Pres Avg (PSIA)"=0.0, "20 Min Pres Avg (PSIA)"=0.0, "25 Min Pres Avg (PSIA)"=0.0, "15 Min Temp Avg (°F) "=0.0, "20 Min Temp Avg (°F)"=0.0, "25 Min Temp Avg (°F)"=0.0, "15 Min Uncorrected Avg (CFH)"=0.0, "20 Min Uncorrected Avg (CFH)"=0.0, "25 Min Uncorrected Avg (CFH)"=0.0, "15 Min Corrected Avg (SCFH)"=0.0, "20 Min Corrected Avg (SCFH)"=0.0, "25 Min Corrected Avg (SCFH)"=0.0, "15 Min Complete"=FALSE, "20 Min Complete"=FALSE, "25 Min Complete"=FALSE, "Heating Value (BTU/ft³)"=0.0, "CO CO2 15 Min"=[], "CO CO2 20 Min"=[], "CO CO2 25 Min"=[], "CO CO2 Real Time"=[]}}, "Threshold Voltage (NI DAQ)"=0.2, "Use RS232 Data Collection"=FALSE, "Use Auto Switching"=FALSE}
  in  "Min to Sec Convert (Total Flow)":dbl=60.0 format="%#_13g"
  in  "Rate Threshold (V)":dbl=0.02
  out "ANSI 1":bool
  out "ANSI 2":bool
  out "ANSI 3":bool
  out "Gas Total Loop":i32
  out "ANSI Loop":i32
  out "Main Control Loop":i32
  out "Debug Array":string[](array[string])
  in  "Debug":bool
  out "Save Loop":i32
  out "Event Loop":i32
  out "Get Gas Data Time":dbl
  out "Data Process Time":dbl
  out "Update Avg Time":dbl
  in  "Inficon Micro GC":T20={"Propane IP Address"="192.168.1.33", "Natural Gas  IP Address"="192.168.1.32", "Remote Port"=502, "Natural Modbus"=refnum, "Propane Modbus"=refnum}
  out "HHV Natural Gas":dbl
  out "HHV Propane":dbl
  out "Num Record":dbl
  # "Meter 1 & 2"
  # "Meter 3 & 4"
  # "Meter 5 & 6"
  # "Heating Value (BTU/ft³)"
  # "Heating Value (BTU/ft³)"
  # "Heating Value (BTU/ft³)"
  # "Custom Commands\nAuthorized ONLY"
  # "Operation Steps:\n\n1) Select Flowmeter Bank\n\n2) Set Heating Value on relevant tab\n\n3) Verify the relevant tab is operating correctly (flow rate from tab is collected here)\n\n4) Set Max Angle to Rotate, Angle per Step, and Data Measure Time\n\n5) Enter a Filename Descriptor (time and date will automatically be added to this)\n\n6) Click Measure Valve\n\n7) Wait for Working light to go off indicating test is complete."
  # "Do Not Change!"
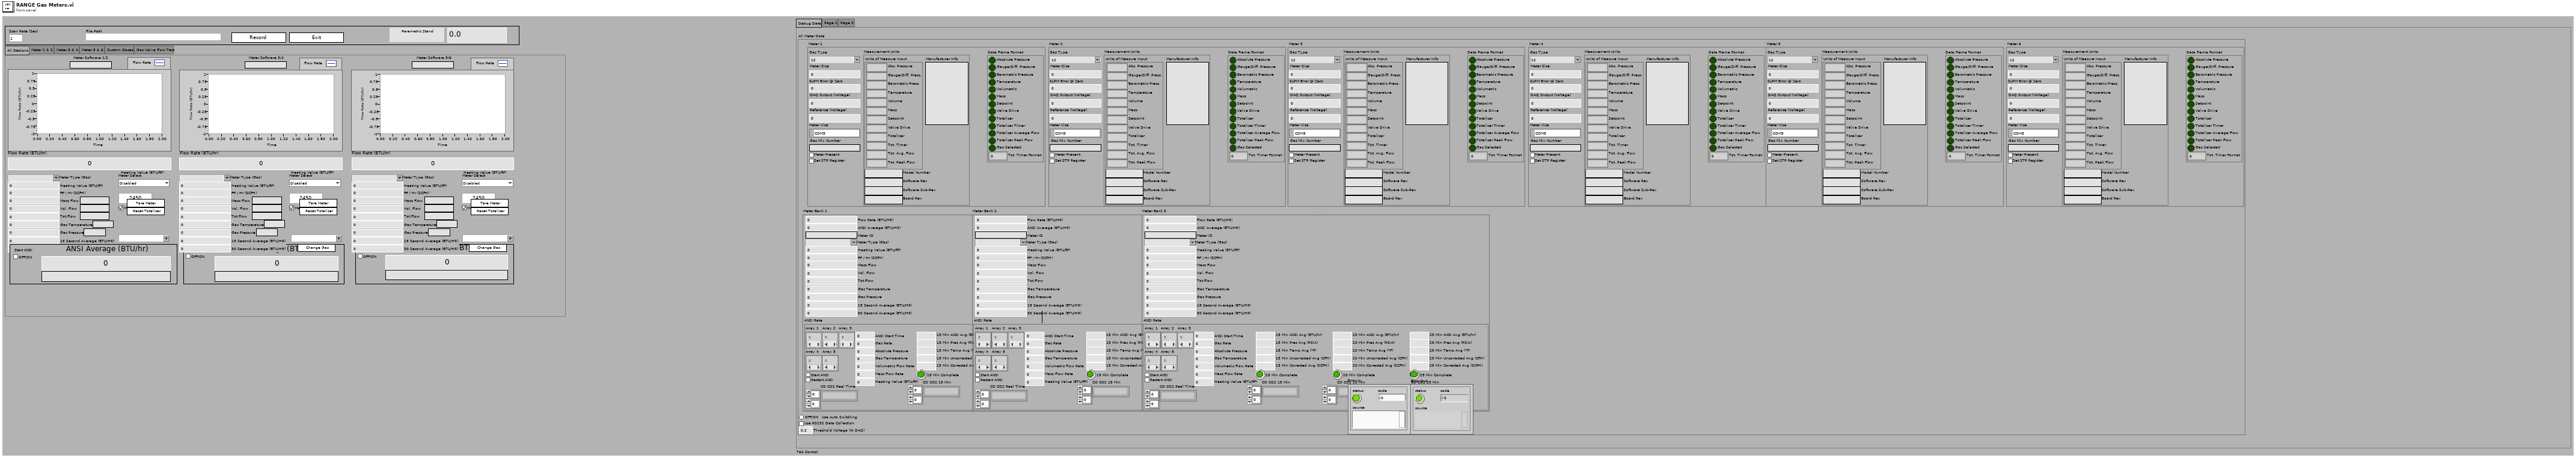
[diagram p1: front panel]
types:
  T1 = typedef "GLVT-Stepper-RotateDirection.ctl" = enum16{"CCW", "CW"}
  T2 = typedef "RANGE Tab Control 2.ctl" = enum32{"All Stations", "Meter 1 & 2", "Meter 3 & 4", "Meter 5 & 6", "Custom Gases", "Gas Valve Flow Test"}
  T3 = typedef "FMA1600A Gas Type.ctl" = string
  T4 = typedef "RANGE Meter Selector 1-2.ctl" = enum16{"Disabled", "Meter 1", "Meter 2", "Auto"}
  T5 = typedef "RANGE Meter Selector 3-4.ctl" = enum16{"Disabled", "Meter 3", "Meter 4", "Auto"}
  T6 = typedef "RANGE Meter Selector 5-6.ctl" = enum16{"Disabled", "Meter 5", "Meter 6", "Auto"}
  T7 = typedef "RANGE Panel Data.ctl" = cluster{"Meter Type (Gas)":T3, "Heating Value (BTU/ft³)":dbl, "Ft³ / Hr (SCFH)":dbl, "15 Second Average (BTU/HR)":dbl, "30 Second Average (BTU/HR)":dbl, "Mass Flow":dbl, "Vol. Flow":dbl, "Gas Temperature":dbl, "Gas Pressure":dbl, "Tot.Flow":dbl}
  T8 = cluster{"Meter Type (Gas)":T3, "Heating Value (BTU/ft³)":dbl, "Ft³ / Hr (SCFH)":dbl, "15 Second Average (BTU/HR)":dbl, "30 Second Average (BTU/HR)":dbl, "Mass Flow":dbl, "Vol. Flow":dbl, "Gas Temperature":dbl, "Gas Pressure":dbl, "Tot.Flow":dbl}
  T9 = enum32{"General Gases", "Pure Non-Corrosice Gases", "Pure Corrosive", "Refrigerants", "Welding Gases", "BioReactor Gases", "Breathing Gases", "Fuel Gases", "Laser Gases", "Create Gas Mixture"}
  T10 = typedef "FMA1600A Commands.ctl" = string
  T11 = typedef "GLVT-Stepper-EnableState.ctl" = enum16{"Enable", "Disable"}
  T12 = typedef "GLVT-FlowmeterBankSelection.ctl" = enum16{"Meter 1 & 2", "Meter 3 & 4", "Meter 5 & 6"}
  T13 = typedef "RANGE DAQ Data Four Meters.ctl" = cluster{"Meter 1":T14, "Meter 2":T14, "Meter 3":T14, "Meter 4":T14, "Meter 5":T14, "Meter 6":T14, "Meter Bank 1":T18, "Meter Bank 2":T18, "Meter Bank 3":T18, "Threshold Voltage (NI DAQ)":dbl, "Use RS232 Data Collection":bool, "Use Auto Switching":bool}
  T14 = typedef "RANGE DAQ Data.ctl" = cluster{"Meter Size":dbl, "DAQ Output (Voltage)":dbl, "Reference (Voltage)":dbl, "Meter Present":bool, "Meter Visa":refnum<visa-resource-name>, "Gas Type":T3, "SLPM Error @ Zero":dbl, "Gas Mix Number":string, "Set STP Register":bool, "Measurement Units":T15, "Data Frame Format":T17}
  T15 = typedef "FMA1600A Units String.ctl" = cluster{"Software Rev":string, "Model Number":string, "Manufacturer Info":string, "Software Sub-Rev":string, "Board Rev":string, "Units of Measure Input":T16}
  T16 = typedef "Units of Measure.ctl" = cluster{"Abs. Pressure":string, "Gauge/Diff. Press.":string, "Barometric Press.":string, "Temperature":string, "Volume":string, "Mass":string, "Setpoint":string, "Valve Drive":string, "Totalizer":string, "Tot. Timer":string, "Tot. Avg. Flow":string, "Tot. Peak Flow":string}
  T17 = typedef "Data Frame.ctl" = cluster{"Absolute Pressure":bool, "Gauge/Diff. Pressure":bool, "Barometric Pressure":bool, "Temperature":bool, "Volumetric":bool, "Mass":bool, "Setpoint":bool, "Valve Drive":bool, "Totalizer":bool, "Totalizer Timer":bool, "Totalizer Average Flow":bool, "Totalizer Peak Flow":bool, "Gas Selected":bool, "Tot. Timer Format":u16}
  T18 = typedef "RANGE GAS Data.ctl" = cluster{"Flow Rate (BTU/HR)":dbl, "ANSI Average (BTU/HR)":dbl, "Panel Data":T7, "Meter ID":string, "ANSI Rate":T19}
  T19 = typedef "RANGE ANSI Rate.ctl" = cluster{"Array 1":dbl[], "Array 3":dbl[], "Array 2":dbl[], "Start ANSI":bool, "ANSI Start Time":dbl, "Restart ANSI":bool, "15 Min ANSI Avg (BTU/hr)":dbl, "20 Min ANSI Avg (BTU/hr)":dbl, "25 Min ANSI Avg (BTU/hr)":dbl, "Absolute Pressure":dbl, "Gas Temperature":dbl, "Volumetric Flow Rate":dbl, "Mass Flow Rate":dbl, "Array 4":dbl[], "Array 5":dbl[], "Gas Rate":dbl, "15 Min Pres Avg (PSIA)":dbl, "20 Min Pres Avg (PSIA)":dbl, "25 Min Pres Avg (PSIA)":dbl, "15 Min Temp Avg (°F) ":dbl, "20 Min Temp Avg (°F)":dbl, "25 Min Temp Avg (°F)":dbl, "15 Min Uncorrected Avg (CFH)":dbl, "20 Min Uncorrected Avg (CFH)":dbl, "25 Min Uncorrected Avg (CFH)":dbl, "15 Min Corrected Avg (SCFH)":dbl, "20 Min Corrected Avg (SCFH)":dbl, "25 Min Corrected Avg (SCFH)":dbl, "15 Min Complete":bool, "20 Min Complete":bool, "25 Min Complete":bool, "Heating Value (BTU/ft³)":dbl, "CO CO2 15 Min":string[][], "CO CO2 20 Min":string[][], "CO CO2 25 Min":string[][], "CO CO2 Real Time":string[][]}
  T20 = typedef "Inficon IP Address.ctl" = cluster{"Propane IP Address":string, "Natural Gas  IP Address":string, "Remote Port":u16, "Natural Modbus":refnum<class "Modbus Master.lvclass">, "Propane Modbus":refnum<class "Modbus Master.lvclass">}
  T21 = typedef "GLVT-States.ctl" = enum16{"Idle", "Initialize", "Read Data", "Next Valve Pos", "Rotate Valve", "Save Data", "Exit"}
  T22 = typedef "UTILITY Notifier.ctl" = enum16{"Set", "Read", "Release Ref"}
  T23 = enum8{"Enabled", "Disabled", "Disabled and Grayed Out"}
  T24 = typedef "FileVersionInformation.ctl" = cluster{"FileVersion":string, "ProductName":string, "InternalName":string, "CompanyName":string, "LegalCopyright":string, "FileDescription":string}
  T25 = typedef "GLVT-FGV-States.ctl" = enum16{"Get", "Set"}
  T26 = enum32{"invalid app kind", "Development System", "Run Time System", "Student Edition", "Embedded LabVIEW", "Evaluation", "Custom"}
  T27 = enum32{"Invalid", "Standard", "Closed", "Hidden", "Minimized", "Maximized"}
  T28 = typedef "Range Meter Bank.ctl" = enum16{"Meter Bank 1", "Meter Bank 2", "Meter Bank 3"}
  T29 = cluster{"Core":cluster{"Current VI Reference":refnum<vi>, "Close Panel on Exit?":bool}, "Bank 1 Counter":i32, "Bank 2 Counter":i32, "Bank 3 Counter":i32, "Meter Data":T13, "File Path":path, "Start Data Save":bool, "Elapsed Time DAQ":dbl}
  T30 = cluster{"Current VI Reference":refnum<vi>, "Close Panel on Exit?":bool}
  T31 = typedef "Inficon Data.ctl" = cluster{"Gross Heating Value, Vol (Real, Dry)":dbl, "Nitrogen Component Normalized Mole % (Dry)":dbl, "Methane Component Normalized Mole % (Dry)":dbl, "Carbon Dioxide Component Normalized Mole % (Dry)":dbl, "Ethane Component Normalized Mole % (Dry)":dbl, "Propane Component Normalized Mole % (Dry)":dbl, "i-Pentane Component Normalized Mole % (Dry)":dbl, "i-Butane Component Normalized Mole % (Dry)":dbl, "n-Butane Component Normalized Mole % (Dry)":dbl, "n-Pentane Component Normalized Mole % (Dry)":dbl, "Hexane Component Normalized Mole % (Dry)":dbl, "Heptane Component Normalized Mole % (Dry)":dbl, "Gross Wobbe Index, Real(Dry)":dbl, "Relative Density, Real(Dry)":dbl, "Propylene Component Normalized Mole % (Dry)":dbl, "C4 Olefins Component Normalized Mole % (Dry)":dbl, "Water Component Normalized Mole % (Dry)":dbl, "Gross Heating Value, Vol (Real, Sat)":dbl, "Natural Gas Data":string[][], "Propane Data":string[][]}
  T32 = typedef "Custom Pallet DBL.ctl" = dbl
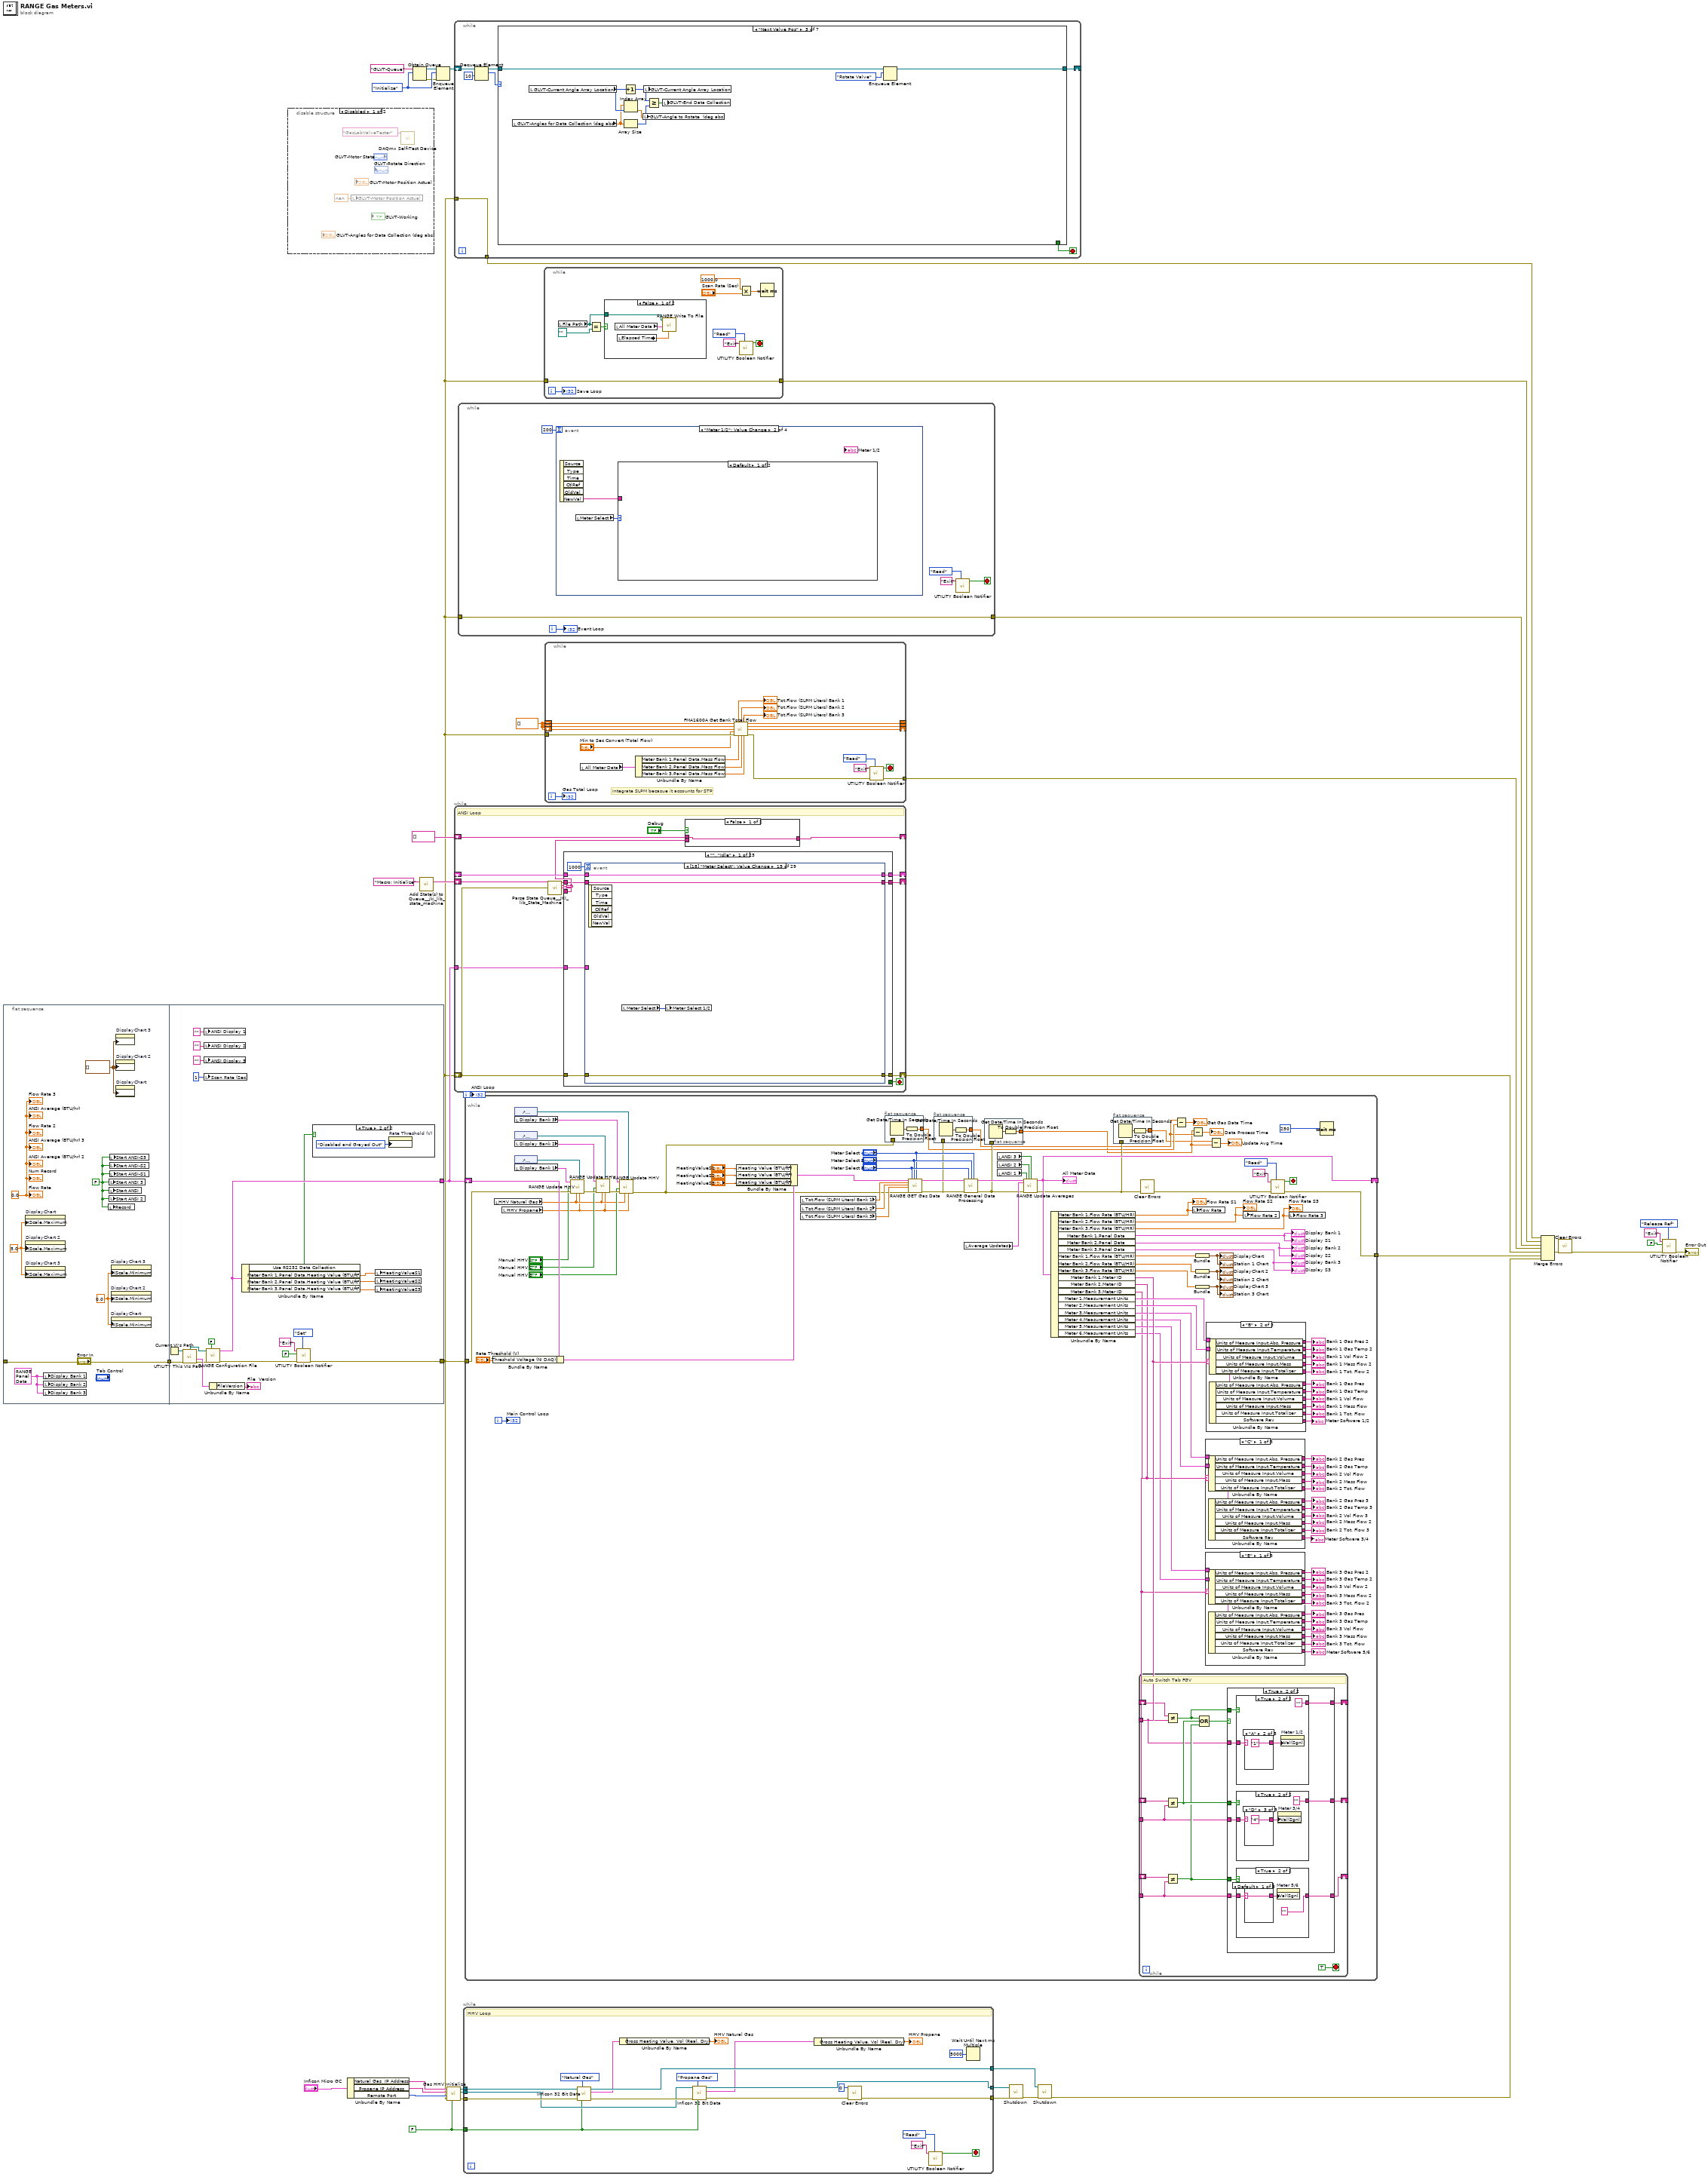
[diagram p0: block diagram]
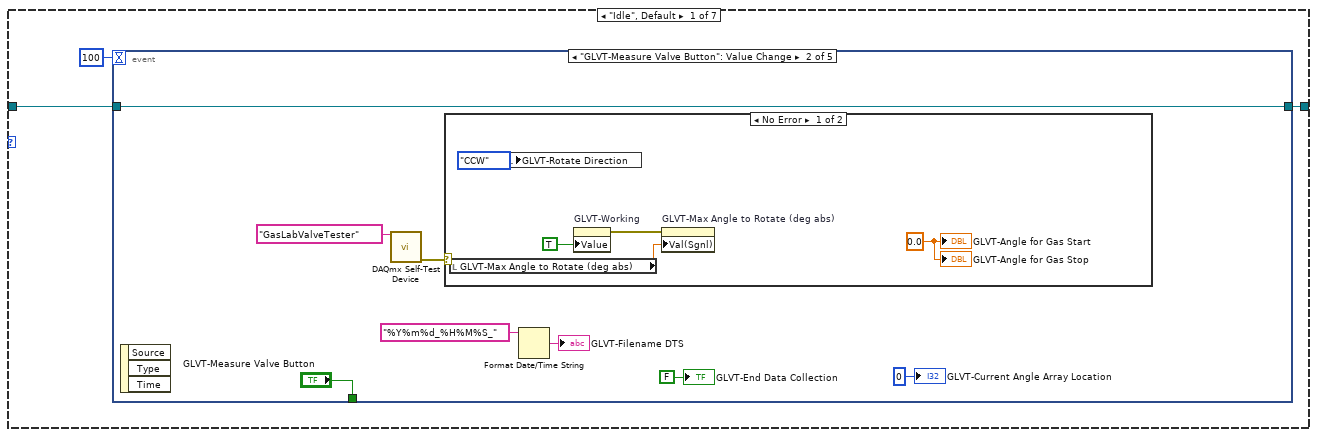
[diagram p2: hidden frame]
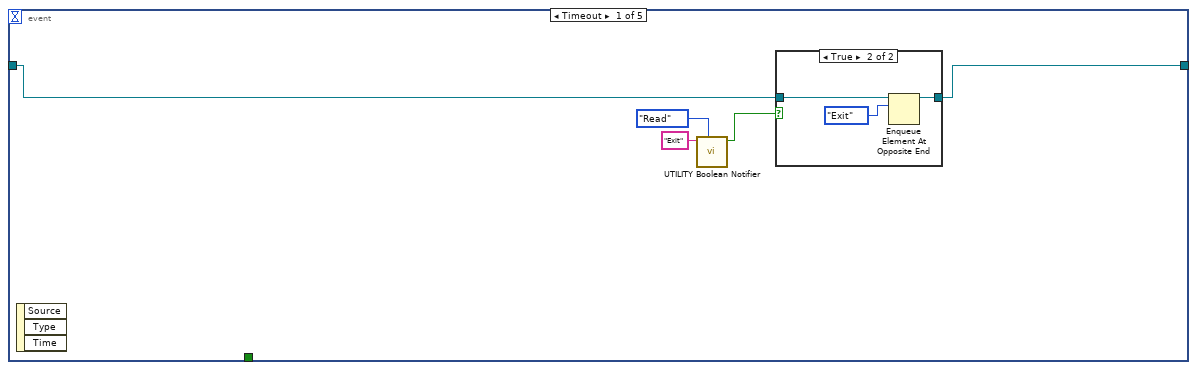
[diagram p3: hidden frame]
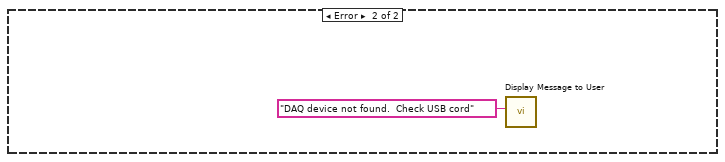
[diagram p5: hidden frame]
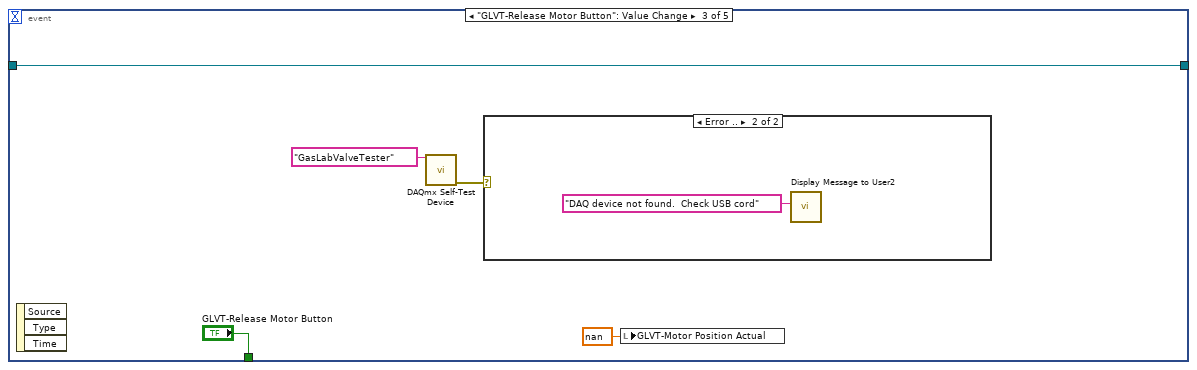
[diagram p6: hidden frame]
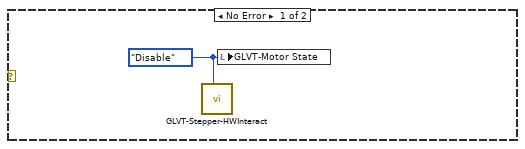
[diagram p7: hidden frame]
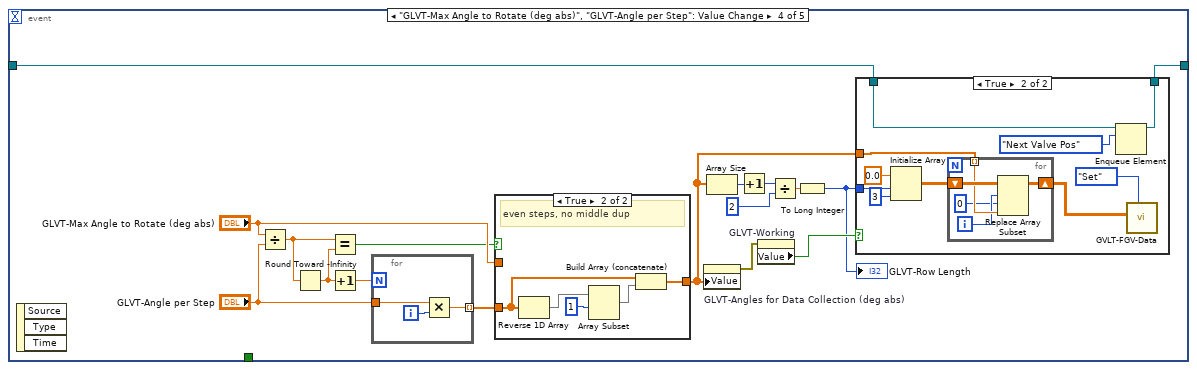
[diagram p8: hidden frame]
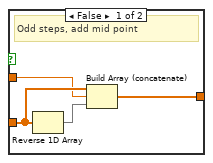
[diagram p10: hidden frame]
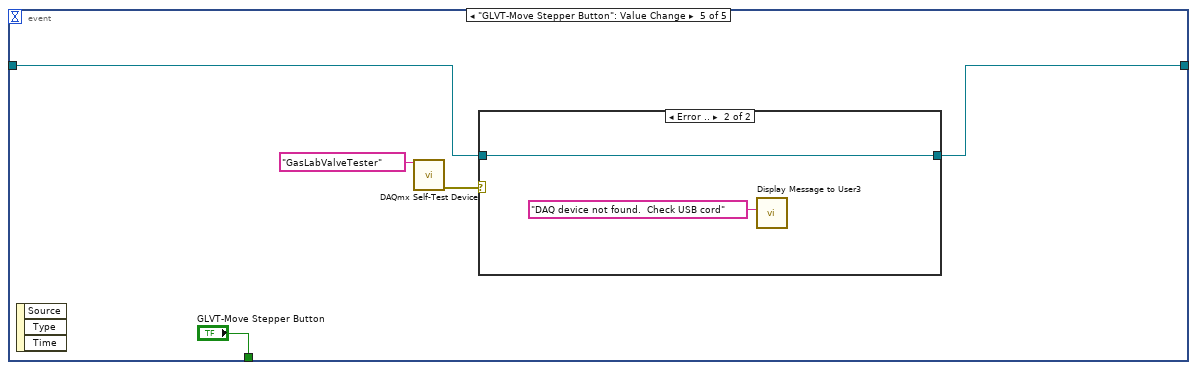
[diagram p11: hidden frame]
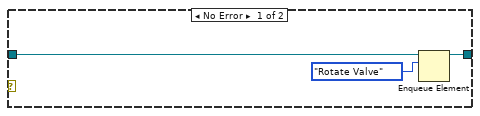
[diagram p12: hidden frame]
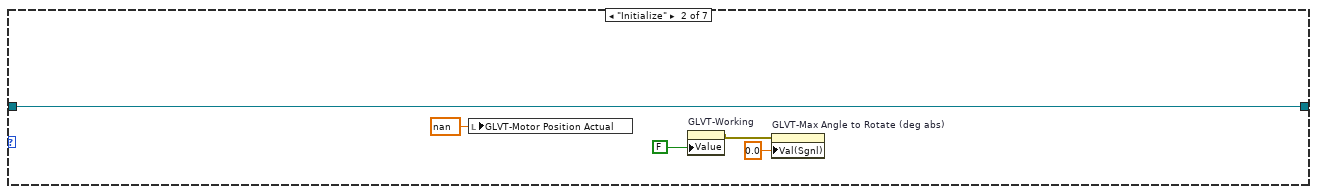
[diagram p13: hidden frame]
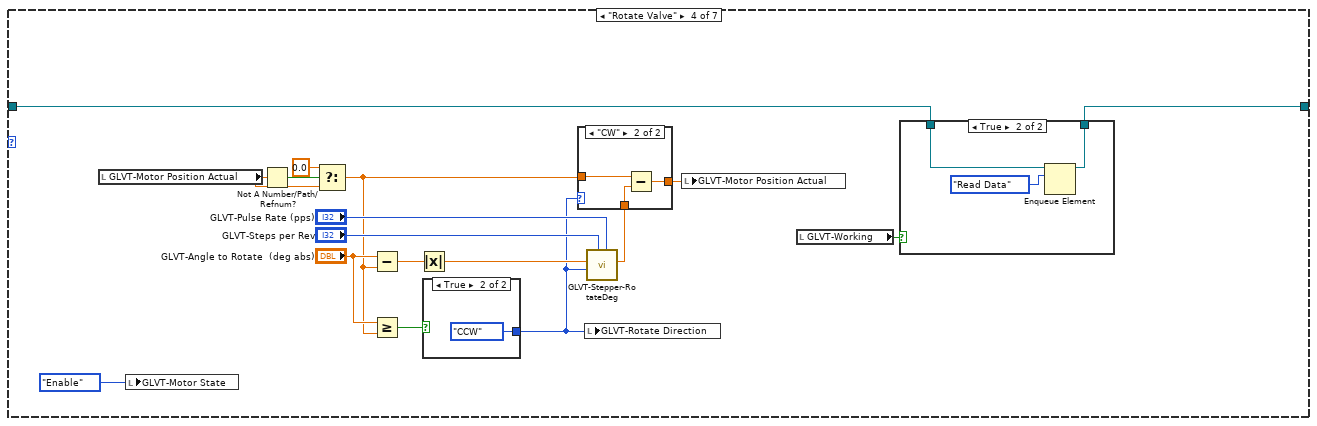
[diagram p14: hidden frame]
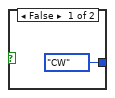
[diagram p16: hidden frame]
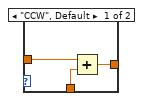
[diagram p17: hidden frame]
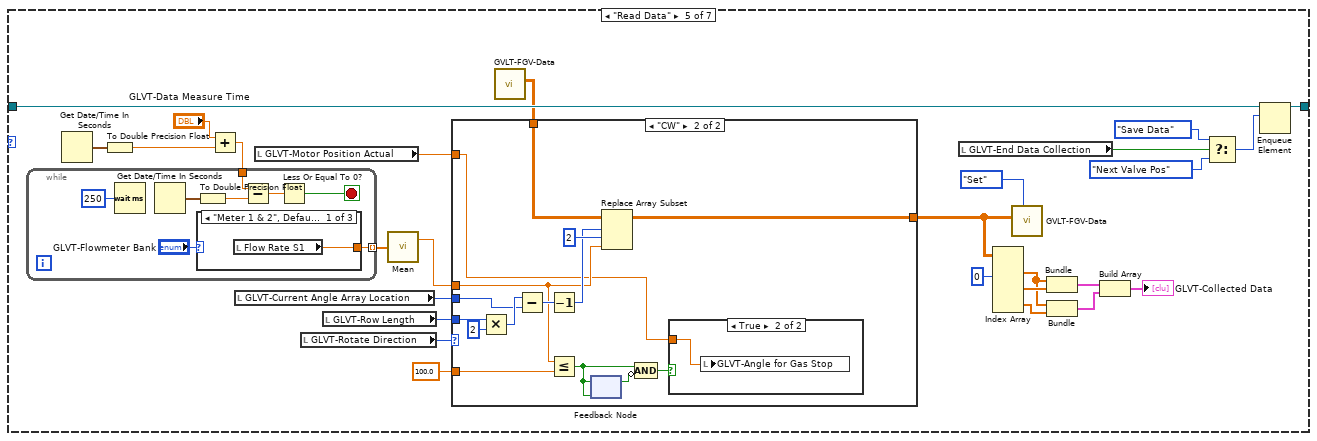
[diagram p18: hidden frame]
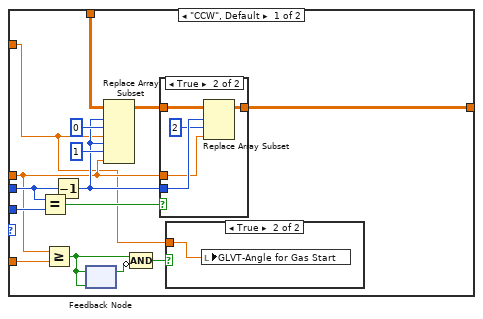
[diagram p19: hidden frame]
diagram:
  w2 = FALSE ("HHV Manual Mode?")
  w20 = GLVT-States."Initialize"
  w32 = dbl[] []
  n1 = flat-sequence {
    tunnel: "Error In" -> [w40]
    tunnel: [w40] -> w37
    tunnel: w37 -> [w63]
    tunnel: [w47] -> w1
    tunnel: [w60] -> w31
    frame #0 {
      w41 = 5.0
      w42 = 0.0
      w39 = FALSE
      w43 = T7 {"Meter Type (Gas)"="", "Heating Value (BTU/ft³)"=0.0, "Ft³ / Hr (SCFH)"=0.0, "15 Second Average (BTU/HR)"=0.0, "30 Second Average (BTU/HR)"=0.0, "Mass Flow"=0.0, "Vol. Flow"=0.0, "Gas Temperature"=0.0, "Gas Pressure"=0.0, "Tot.Flow"=0.0} ("Display Bank 1")
      w44 = 0.0
      w45 = cluster{"[0]":dbl}[] []
      n2 = property on="DisplayChart" class="WFChart (strict)"("XScale.Maximum"=w41) -> ()  [unwired: 2 in, 2 out]
      n3 = property on="DisplayChart 2" class="WFChart (strict)"("XScale.Maximum"=w41) -> ()  [unwired: 2 in, 2 out]
      n4 = property on="DisplayChart 3" class="WFChart (strict)"("XScale.Maximum"=w41) -> ()  [unwired: 2 in, 2 out]
      n5 = local write "Display Bank 1"(w43) -> ()
      n6 = local write "Display Bank 2"(w43) -> ()
      n7 = local write "Display Bank 3"(w43) -> ()
      n8 = local write "Record"(w39) -> ()
      n9 = local write "Start ANSI 3"(w39) -> ()
      n10 = local write "Start ANSI"(w39) -> ()
      n11 = local write "Start ANSI 2"(w39) -> ()
      n12 = local write "Start ANSI-S3"(w39) -> ()
      n13 = local write "Start ANSI-S2"(w39) -> ()
      n14 = local write "Start ANSI-S1"(w39) -> ()
      n15 = property on="DisplayChart 3" class="WFChart (strict)"("XScale.Minimum"=w42) -> ()  [unwired: 2 in, 2 out]
      n16 = property on="DisplayChart 2" class="WFChart (strict)"("XScale.Minimum"=w42) -> ()  [unwired: 2 in, 2 out]
      n17 = property on="DisplayChart" class="WFChart (strict)"("XScale.Minimum"=w42) -> ()  [unwired: 2 in, 2 out]
      n18 = property on="DisplayChart 3" class="WFChart (strict)"("History Data"=w45) -> ()  [unwired: 2 in, 2 out]
      n19 = property on="DisplayChart 2" class="WFChart (strict)"("History Data"=w45) -> ()  [unwired: 2 in, 2 out]
      n20 = property on="DisplayChart" class="WFChart (strict)"("History Data"=w45) -> ()  [unwired: 2 in, 2 out]
      "Num Record" <- w44
      "ANSI Average (BTU/hr)" <- w44
      "Flow Rate" <- w44
      "Flow Rate 2" <- w44
      "ANSI Average (BTU/hr) 2" <- w44
      "Flow Rate 3" <- w44
      "ANSI Average (BTU/hr) 3" <- w44
    }
    frame #1 {
      n21 = Current VI's Path() -> (path=w66:path)
      n22 = call "UTILITY This VIs Path.vi"("path"=w66, "error in (no error)"=w63) -> ("Folder Path"=w58:path, "FileVersionInfo Out"=w65:T24, "error out"=w62:errorcluster)  [unwired: 7 in, 4 out]
      n23 = local write "ANSI Display 1"("" ("ANSI Display 1")) -> ()
      n24 = local write "ANSI Display 2"("" ("ANSI Display 2")) -> ()
      n25 = local write "ANSI Display 3"("" ("ANSI Display 3")) -> ()
      n26 = local write "Scan Rate (Sec)"(1 ("Scan Rate (Sec)")) -> ()
      n27 = call "RANGE Configuration File.vi"("Debug"=FALSE, "Error In"=w62, "Gas Lab Config File"=w58) -> ("Error Out"=w48:errorcluster, "Meter Data"=w60:T13)  [unwired: 7 in]
      n28 = Unbundle By Name(w65) -> ("FileVersion"=→"File  Version":string)
      n29 = Unbundle By Name(w60) -> ("Use RS232 Data Collection"=w59:bool, "Meter Bank 1.Panel Data.Heating Value (BTU/ft³)"=w54:dbl, "Meter Bank 2.Panel Data.Heating Value (BTU/ft³)"=w53:dbl, "Meter Bank 3.Panel Data.Heating Value (BTU/ft³)"=w52:dbl)
      n30 = call "UTILITY Boolean Notifier.vi"("Status"=UTILITY_Notifier."Set", "error in (no error)"=w48, "Set Status"=FALSE, "name (unnamed)"="Exit") -> ("error out"=w47:errorcluster)  [unwired: 6 in, 1 out]
      n31 = case shown="True" w59 {
        frame False {
          n32 = property on="Rate Threshold (V)" class="DigNum (strict)"("DisabledEnum"=T23."Enabled" ("Disabled")) -> ()  [unwired: 2 in, 2 out]
        }
        frame True {
          n33 = property on="Rate Threshold (V)" class="DigNum (strict)"("DisabledEnum"=T23."Disabled and Grayed Out" ("Disabled")) -> ()  [unwired: 2 in, 2 out]
        }
      }
      n34 = local write "HeatingValueS1"(w54) -> ()
      n35 = local write "HeatingValueS2"(w53) -> ()
      n36 = local write "HeatingValueS3"(w52) -> ()
    }
  }
  n37 = disable-structure shown="Disabled" {
    frame Disabled {
      n38 = local write "GLVT-Motor Position Actual"(nan ("Motor Position")) -> ()
      n39 = call <vilib>:"DAQmx Self-Test Device.vi"("device in"=tag "GasLabValveTester") -> ()  [unwired: 14 in, 1 out]
    }
    frame Enabled {
    }
  }
  n40 = Unbundle By Name("Inficon Micro GC") -> ("Natural Gas  IP Address"=w11:string, "Propane IP Address"=w10:string, "Remote Port"=w9:u16)
  n41 = Obtain Queue(name (unnamed)="GLVT-Queue", element data type=w20) -> (queue out=w19:refnum<queue>, error out=w18:errorcluster)  [unwired: 3 in, 1 out]
  n42 = call <vilib>:"Add State(s) to Queue__jki_lib_state_machine.vi"("State(s) in (\"\")"="Macro: Initialize") -> ("States Out"=w36:string)  [unwired: 14 in]
  n43 = Enqueue Element(queue=w19, element=w20, error in (no error)=w18) -> (queue out=w21:refnum<queue>)  [unwired: 1 in, 2 out]
  n44 = call "Gas HHV Initialize.vi"("Manual HHV Mode?"=w2, "error in (no error)"=w1, "Remote Port"=w9, "Propane IP Address"=w10, "Natural Gas  IP Address"=w11) -> ("error out"=w8:errorcluster, "Propane Modbus"=w6:refnum<class "Modbus Master.lvclass">, "Natural Modbus"=w7:refnum<class "Modbus Master.lvclass">)  [unwired: 4 in]
  n45 = while {
    shift-right: [w73] -> _
    shift-left: w21 -> [w76]
    tunnel: w1 -> [w71]
    tunnel: [w71] -> w16
    stop <- w77 stop-if-true
    n46 = Dequeue Element(queue=w76, timeout in ms (-1)=10) -> (queue out=w75:refnum<queue>, element=w74:T21)  [unwired: 1 in, 2 out]
    n47 = case shown="\"Next Valve Pos\"" w74 {
      tunnel: [_ _ _ _ _ _ TRUE] -> w77
      tunnel: w75 -> [w79 w170 w179 w182 w235 w314 w322]
      tunnel: [w78 w170 w172 w181 w234 w314 w322] -> w73
      frame "Idle", Default {
        n48 = event shown="[1] \"GLVT-Measure Valve Button\": Value Change" {
          selector: _ -> [_ _ _ _ _]
          dyn-events: _ -> [_ _ _ _ _]
          timeout: 100 -> [_ _ _ _ _]
          tunnel: w79 -> [w84 w97 w108 w118 w160]
          tunnel: [w85 w97 w108 w117 w158] -> w78
          tunnel: [_ "GLVT-Measure Valve Button" "GLVT-Release Motor Button" _ "GLVT-Move Stepper Button"] -> _
          event Timeout {
            n49 = event-data() -> ()  [unwired: 1 in, 3 out]
            n50 = call "UTILITY Boolean Notifier.vi"("Status"=UTILITY_Notifier."Read", "name (unnamed)"="Exit") -> ("latest READ notification"=w81:bool)  [unwired: 8 in, 1 out]
            n51 = case shown="True" w81 {
              tunnel: [w86 w88] -> w85
              tunnel: w84 -> [w86 w87]
              frame False {
              }
              frame True {
                n52 = Enqueue Element At Opposite End(queue=w87, element=GLVT-States."Exit") -> (queue out=w88:refnum<queue>)  [unwired: 2 in, 2 out]
              }
            }
          }
          event "GLVT-Measure Valve Button": Value Change {
            n53 = event-data() -> ()  [unwired: 1 in, 3 out]
            n54 = call <vilib>:"DAQmx Self-Test Device.vi"("device in"=tag "GasLabValveTester") -> ("error out"=w90:errorcluster)  [unwired: 14 in]
            n55 = case shown="No Error" w90 {
              frame No Error {
                w98 = 0.0 ("Angle for Gas Start")
                n56 = local read "GLVT-Max Angle to Rotate (deg abs)"() -> (w102:dbl)
                n57 = local write "GLVT-Rotate Direction"(GLVT-Stepper-RotateDirection."CCW" ("Rotate Direction")) -> ()
                n58 = property on="GLVT-Working" class="Bool (strict)"("Value"=TRUE ("Working")) -> (error out=w100:errorcluster)  [unwired: 2 in, 1 out]
                n59 = property on="GLVT-Max Angle to Rotate (deg abs)" class="DigNum (strict)"(error in=w100, "Val(Sgnl)"=w102) -> ()  [unwired: 1 in, 2 out]
                "GLVT-Angle for Gas Start" <- w98
                "GLVT-Angle for Gas Stop" <- w98
              }
              frame Error {
                n60 = call "Display Message to User"("Message"="DAQ device not found.  Check USB cord") -> ()  [unwired: 9 in, 2 out]
              }
            }
            n61 = Format Date/Time String(time format string (%c)="%Y%m%d_%H%M%S_") -> (date/time string=→"GLVT-Filename DTS":string)  [unwired: 2 in]
            "GLVT-Current Angle Array Location" <- 0 ("Current Angle Array Location")
            "GLVT-End Data Collection" <- FALSE ("End Data Collection")
          }
          event "GLVT-Release Motor Button": Value Change {
            n62 = event-data() -> ()  [unwired: 1 in, 3 out]
            n63 = call <vilib>:"DAQmx Self-Test Device.vi"("device in"=tag "GasLabValveTester") -> ("error out"=w104:errorcluster)  [unwired: 14 in]
            n64 = case shown="Error .." w104 {
              frame No Error {
                w109 = GLVT-Stepper-EnableState."Disable" ("GLVT-Enable State")
                n65 = call "GLVT-Stepper-HWInteract.vi"("GLVT-Enable State"=w109) -> ()  [unwired: 10 in, 1 out]
                n66 = local write "GLVT-Motor State"(w109) -> ()
              }
              frame Error {
                n67 = call "Display Message to User2"("Message"="DAQ device not found.  Check USB cord") -> ()  [unwired: 9 in, 2 out]
              }
            }
            n68 = local write "GLVT-Motor Position Actual"(nan ("Motor Position")) -> ()
          }
          event "GLVT-Max Angle to Rotate (deg abs)", "GLVT-Angle per Step": Value Change {
            n69 = event-data() -> ()  [unwired: 1 in, 3 out]
            n70 = Divide(x="GLVT-Max Angle to Rotate (deg abs)", y="GLVT-Angle per Step") -> (x/y=w123:dbl)
            n71 = Round Toward -Infinity(1:w123) -> (0:w122:dbl)
            n72 = Equal?(x=w123, y=w122) -> (x = y?=w121:bool)
            n73 = Increment(x=w122) -> (x+1=w127:dbl)
            n74 = for {
              N: w127 -> [_]
              tunnel: "GLVT-Angle per Step" -> [w154]
              tunnel: [w153] -> w125 mode=indexing
              i -> [w155]
              n75 = Multiply(x=w154, y=w155) -> (x*y=w153:dbl)
            }
            n76 = case shown="True" w121 {
              tunnel: [w147 w148] -> w111
              tunnel: w125 -> [w146 w149]
              tunnel: "GLVT-Max Angle to Rotate (deg abs)" -> [w144 _]
              frame False {
                # "Odd steps, add mid point"
                n77 = Reverse 1D Array(array=w146) -> (reversed array=w145:dbl[])
                n78 = Build Array (concatenate)(w146, w144, w145) -> (w147:dbl[])
              }
              frame True {
                # "even steps, no middle dup"
                n79 = Reverse 1D Array(array=w149) -> (reversed array=w152:dbl[])
                n80 = Array Subset(array=w152, index=1) -> (w150:dbl[])  [unwired: 1 in]
                n81 = Build Array (concatenate)(w149, w150) -> (w148:dbl[])
              }
            }
            n82 = property on="GLVT-Angles for Data Collection (deg abs)" class="Arr (strict)"("Value"=w111) -> (error out=w120:errorcluster)  [unwired: 2 in, 1 out]
            n83 = Array Size(array=w111) -> (size(s)=w116:i32)
            n84 = Increment(x=w116) -> (x+1=w115:i32)
            n85 = property on="GLVT-Working" class="Bool (strict)"(error in=w120) -> ("Value"=w119:bool)  [unwired: 1 in, 2 out]
            n86 = Divide(x=w115, y=2) -> (x/y=w113:dbl)
            n87 = To Long Integer(number=w113) -> (32bit integer=w112:i32)
            "GLVT-Row Length" <- w112
            n88 = case shown="True" w119 {
              tunnel: [w128 w137] -> w117
              tunnel: w118 -> [w128 w138]
              tunnel: w112 -> [_ w135]
              tunnel: w111 -> [_ w130]
              frame False {
              }
              frame True {
                n89 = Initialize Array(0.0 ("element"), w135, 3 ("dimension size")) -> (w131:dbl[][])
                n90 = for {
                  tunnel: w130 -> [w142] mode=indexing
                  shift-right: [w139] -> w129
                  shift-left: w131 -> [w143]
                  i -> [w141]
                  n91 = Replace Array Subset(array=w143, new element=w142, index (row)=w141, index (col)=0 ("disabled index (col)")) -> (w139:dbl[][])
                }
                n92 = Enqueue Element(queue=w138, element=GLVT-States."Next Valve Pos") -> (queue out=w137:refnum<queue>)  [unwired: 2 in, 2 out]
                n93 = call "GVLT-FGV-Data.vi"("State"=GLVT-FGV-States."Set", "Data In"=w129) -> ()  [unwired: 8 in, 2 out]
              }
            }
          }
          event "GLVT-Move Stepper Button": Value Change {
            n94 = event-data() -> ()  [unwired: 1 in, 3 out]
            n95 = call <vilib>:"DAQmx Self-Test Device.vi"("device in"=tag "GasLabValveTester") -> ("error out"=w156:errorcluster)  [unwired: 14 in]
            n96 = case shown="Error .." w156 {
              tunnel: w160 -> [w163 w165]
              tunnel: [w162 w165] -> w158
              frame No Error {
                n97 = Enqueue Element(queue=w163, element=GLVT-States."Rotate Valve") -> (queue out=w162:refnum<queue>)  [unwired: 2 in, 2 out]
              }
              frame Error {
                n98 = call "Display Message to User3"("Message"="DAQ device not found.  Check USB cord") -> ()  [unwired: 9 in, 2 out]
              }
            }
          }
        }
      }
      frame "Initialize" {
        n99 = local write "GLVT-Motor Position Actual"(nan ("Motor Position")) -> ()
        n100 = property on="GLVT-Working" class="Bool (strict)"("Value"=FALSE ("Working")) -> (error out=w166:errorcluster)  [unwired: 2 in, 1 out]
        n101 = property on="GLVT-Max Angle to Rotate (deg abs)" class="DigNum (strict)"(error in=w166, "Val(Sgnl)"=0.0 ("Value (Signaling)")) -> ()  [unwired: 1 in, 2 out]
      }
      frame "Next Valve Pos" {
        n102 = local read "GLVT-Angles for Data Collection (deg abs)"() -> (w176:dbl[])
        n103 = local read "GLVT-Current Angle Array Location"() -> (w178:i32)
        n104 = Increment(x=w178) -> (x+1=w174:i32)
        n105 = Index Array(array=w176, index=w178) -> (element=w177:dbl)
        n106 = Array Size(array=w176) -> (size(s)=w175:i32)
        n107 = local write "GLVT-Angle to Rotate  (deg abs)"(w177) -> ()
        n108 = local write "GLVT-Current Angle Array Location"(w174) -> ()
        n109 = Greater Or Equal?(x=w174, y=w175) -> (x >= y?=w173:bool)
        n110 = local write "GLVT-End Data Collection"(w173) -> ()
        n111 = Enqueue Element(queue=w179, element=GLVT-States."Rotate Valve") -> (queue out=w172:refnum<queue>)  [unwired: 2 in, 2 out]
      }
      frame "Rotate Valve" {
        n112 = local read "GLVT-Motor Position Actual"() -> (w190:dbl)
        n113 = local write "GLVT-Motor State"(GLVT-Stepper-EnableState."Enable" ("GLVT-Enable State")) -> ()
        n114 = Not A Number/Path/Refnum?(number/path/refnum=w190) -> (NaN/Path/Refnum?=w191:bool)
        n115 = Select(t=0.0, s=w191, f=w190) -> (s? t:f=w187:dbl)
        n116 = Subtract(x="GLVT-Angle to Rotate  (deg abs)", y=w187) -> (x-y=w186:dbl)
        n117 = Greater Or Equal?(x="GLVT-Angle to Rotate  (deg abs)", y=w187) -> (x >= y?=w189:bool)
        n118 = Absolute Value(x=w186) -> (abs(x)=w185:dbl)
        n119 = case shown="True" w189 {
          tunnel: [GLVT-Stepper-RotateDirection."CW" ("Rotate Direction") GLVT-Stepper-RotateDirection."CCW" ("Rotate Direction")] -> w180
          frame False {
          }
          frame True {
          }
        }
        n120 = local write "GLVT-Rotate Direction"(w180) -> ()
        n121 = call "GLVT-Stepper-RotateDeg.vi"("Pulse Rate (pps)"="GLVT-Pulse Rate (pps)", "Steps per Rev"="GLVT-Steps per Rev", "Rotate Direction"=w180, "Rotation Angle (deg)"=w185) -> ("Actual Rotation Angle (deg)"=w196:dbl)  [unwired: 6 in, 1 out]
        n122 = case shown="\"CW\"" w180 {
          tunnel: w187 -> [w205 w208]
          tunnel: w196 -> [w204 w207]
          tunnel: [w203 w206] -> w184
          frame "CCW", Default {
            n123 = Add(x=w205, y=w204) -> (x+y=w203:dbl)
          }
          frame "CW" {
            n124 = Subtract(x=w208, y=w207) -> (x-y=w206:dbl)
          }
        }
        n125 = local write "GLVT-Motor Position Actual"(w184) -> ()
        n126 = local read "GLVT-Working"() -> (w183:bool)
        n127 = case shown="True" w183 {
          tunnel: [w197 w199] -> w181
          tunnel: w182 -> [w197 w200]
          frame False {
          }
          frame True {
            n128 = Enqueue Element(queue=w200, element=GLVT-States."Read Data") -> (queue out=w199:refnum<queue>)  [unwired: 2 in, 2 out]
          }
        }
      }
      frame "Read Data" {
        n129 = Get Date/Time In Seconds() -> (seconds since 1Jan1904=w226:timestamp)
        n130 = To Double Precision Float(number=w226) -> (double precision float=w224:dbl)
        n131 = Add(x="GLVT-Data Measure Time", y=w224) -> (x+y=w223:dbl)
        n132 = while {
          tunnel: w223 -> [w278]
          tunnel: [w275] -> w222 mode=indexing
          stop <- w276 stop-if-true
          n133 = Wait (ms)(milliseconds to wait=u32 250) -> ()  [unwired: 1 out]
          n134 = Get Date/Time In Seconds() -> (seconds since 1Jan1904=w280:timestamp)
          n135 = case shown="\"Meter 1 & 2\", Default" "GLVT-Flowmeter Bank" {
            tunnel: [w282 w283 w284] -> w275
            frame "Meter 1 & 2", Default {
              n136 = local read "Flow Rate S1"() -> (w282:dbl)
            }
            frame "Meter 3 & 4" {
              n137 = local read "Flow Rate S2"() -> (w283:dbl)
            }
            frame "Meter 5 & 6" {
              n138 = local read "Flow Rate S3"() -> (w284:dbl)
            }
          }
          n139 = To Double Precision Float(number=w280) -> (double precision float=w279:dbl)
          n140 = Subtract(x=w278, y=w279) -> (x-y=w277:dbl)
          n141 = Less Or Equal To 0?(x=w277) -> (x <= 0?=w276:bool)
        }
        n142 = local read "GLVT-Current Angle Array Location"() -> (w220:i32)
        n143 = local read "GLVT-Motor Position Actual"() -> (w218:dbl)
        n144 = local read "GLVT-Rotate Direction"() -> (w221:T1)
        n145 = local read "GLVT-Row Length"() -> (w216:i32)
        n146 = call-poly <vilib>:"Mean.vi"("X"=w222) -> ("mean"=w219:dbl)  [unwired: 1 out]
        n147 = call "GVLT-FGV-Data.vi"() -> ("Data Out"=w217:dbl[][])  [unwired: 10 in, 1 out]
        n148 = case shown="\"CW\"" w221 {
          tunnel: w220 -> [w244 w268]
          tunnel: w219 -> [w241 w259]
          tunnel: w218 -> [w237 w258]
          tunnel: w217 -> [w250 w272]
          tunnel: [w243 w265] -> w215
          tunnel: w216 -> [w247 w271]
          tunnel: 100.0 ("y") -> [w236 w261]
          frame "CCW", Default {
            n149 = Equal?(x=w244, y=w247) -> (x = y?=w246:bool)
            n150 = Greater Or Equal?(x=w241, y=w236) -> (x >= y?=w240:bool)
            n151 = Decrement(x=w244) -> (x-1=w242:i32)
            n152 = feedback-in #1(w240) -> ()
            n153 = feedback #1(w240) -> (w239:bool)
            n154 = Replace Array Subset(array=w250, new element #1=w237, index (row) #1=w242, index (col) #1=0 ("disabled index (col)"), new element #2=w241, index (row) #2=w242, index (col) #2=1 ("disabled index (col)")) -> (w245:dbl[][])
            n155 = Compound Arithmetic op=AND(w240, invert w239) -> (w238:bool)
            n156 = case shown="True" w246 {
              tunnel: w245 -> [w252 w257]
              tunnel: w242 -> [_ w256]
              tunnel: w241 -> [_ w254]
              tunnel: [w252 w253] -> w243
              frame False {
              }
              frame True {
                n157 = Replace Array Subset(array=w257, new element=w254, index (row)=w256, index (col)=2 ("disabled index (col)")) -> (w253:dbl[][])
              }
            }
            n158 = case shown="True" w238 {
              tunnel: w237 -> [_ w251]
              frame False {
              }
              frame True {
                n159 = local write "GLVT-Angle for Gas Start"(w251) -> ()
              }
            }
          }
          frame "CW" {
            n160 = Multiply(x=w271, y=2) -> (x*y=w269:i32)
            n161 = Subtract(x=w269, y=w268) -> (x-y=w267:i32)
            n162 = Decrement(x=w267) -> (x-1=w264:i32)
            n163 = Less Or Equal?(x=w259, y=w261) -> (x <= y?=w263:bool)
            n164 = feedback #2(w263) -> (w262:bool)
            n165 = feedback-in #2(w263) -> ()
            n166 = Replace Array Subset(array=w272, new element=w259, index (row)=w264, index (col)=2 ("disabled index (col)")) -> (w265:dbl[][])
            n167 = Compound Arithmetic op=AND(w263, invert w262) -> (w260:bool)
            n168 = case shown="True" w260 {
              tunnel: w258 -> [_ w273]
              frame False {
              }
              frame True {
                n169 = local write "GLVT-Angle for Gas Stop"(w273) -> ()
              }
            }
          }
        }
        n170 = local read "GLVT-End Data Collection"() -> (w233:bool)
        n171 = Index Array(array=w215, index (col) #1=0 ("disabled index (col)")) -> (element #1=w213:dbl[], element #2=w227:dbl[], element #3=w214:dbl[])  [unwired: 5 in]
        n172 = call "GVLT-FGV-Data.vi"("State"=GLVT-FGV-States."Set", "Data In"=w215) -> ()  [unwired: 8 in, 2 out]
        n173 = Bundle("Data Out"=w213, "Data Out"=w227) -> (w212:cluster{"Data Out":dbl[], "Data Out":dbl[]})  [unwired: 1 in]
        n174 = Bundle("Data Out"=w213, "Data Out"=w214) -> (w211:cluster{"Data Out":dbl[], "Data Out":dbl[]})  [unwired: 1 in]
        n175 = Build Array(w212, w211) -> (→"GLVT-Collected Data":cluster{"Data Out":dbl[], "Data Out":dbl[]}[])
        n176 = Select(t=GLVT-States."Save Data" ("element"), s=w233, f=GLVT-States."Next Valve Pos" ("element")) -> (s? t:f=w230:T21)
        n177 = Enqueue Element(queue=w235, element=w230) -> (queue out=w234:refnum<queue>)  [unwired: 2 in, 2 out]
      }
      frame "Save Data" {
        w302 = "," ("delimiter (Tab)")
        n178 = local write "GLVT-Working"(FALSE ("Working")) -> ()
        n179 = local read "GLVT-Filename DTS"() -> (w311:string)
        n180 = call <vilib>:"Check if File or Folder Exists.vi"("path"=path "C:/Gas Flow Meter") -> ("file or folder exists?"=w307:bool, "dup path"=w306:path)  [unwired: 8 in, 1 out]
        n181 = case shown="False" w307 {
          tunnel: w306 -> [w316 w317]
          tunnel: [w315 w317] -> w299
          frame False {
            # "create folder"
            n182 = Create Folder(path (use dialog)=w316) -> (created path=w315:path)  [unwired: 2 in, 2 out]
          }
          frame True {
            # "exists, do nothing"
          }
        }
        n183 = call "GVLT-FGV-Data.vi"() -> ("Data Out"=w305:dbl[][])  [unwired: 10 in, 1 out]
        n184 = local read "GLVT-Angle for Gas Start"() -> (w290:dbl)
        n185 = local read "GLVT-Angle for Gas Stop"() -> (w289:dbl)
        n186 = Concatenate Strings(w311, "GLVT-Filename Descriptor", ".csv" ("string")) -> (w309:string)
        n187 = call <vilib>:"Is Name Multiplatform.vi"("filename"=w309) -> ("suggested filename"=w298:string)  [unwired: 6 in, 4 out]
        n188 = Array To Spreadsheet String(delimiter (Tab)=w302, array=string[] ["Angle", "Flow Rate (CCW)", "Flow Rate (CW)", "Gas Start Angle", "Gas Stop Angle"], 3:"%s" ("format string")) -> (spreadsheet string=w300:string)
        n189 = Array To Spreadsheet String(delimiter (Tab)=w302, array=w305, 3:"%0.3f" ("format string")) -> (spreadsheet string=w292:string)
        n190 = Search/Split String(string=w292, search string/char (-)="\r\n") -> (substring before match=w291:string, match + rest of string=w286:string)  [unwired: 1 in, 1 out]
        n191 = Format Into String(format string=",%0.3f,%0.3f", w290, w289) -> (resulting string=w287:string)  [unwired: 2 in, 1 out]
        n192 = Concatenate Strings(w291, w287, w286) -> (w285:string)
        n193 = Build Path(base path=w299, name or relative path=w298) -> (appended path=w294:path)
        "GLVT-Save Data Location" <- w294
        n194 = Concatenate Strings(w300, w285) -> (w297:string)
        n195 = Write to Text File(file (use dialog)=w294, text=w297) -> (refnum out=w295:refnum<file>, error out=w296:errorcluster)  [unwired: 2 in, 1 out]
        n196 = Close File(refnum=w295, error in=w296) -> ()  [unwired: 2 out]
      }
      frame "Exit" {
        n197 = local write "GLVT-Motor Position Actual"(nan ("Motor Position")) -> ()
        n198 = local write "GLVT-Working"(FALSE ("Working")) -> ()
        n199 = call <vilib>:"DAQmx Self-Test Device.vi"("device in"=tag "GasLabValveTester") -> ("error out"=w318:errorcluster)  [unwired: 14 in]
        n200 = case shown="Error .." w318 {
          frame No Error {
            w324 = GLVT-Stepper-EnableState."Disable" ("GLVT-Enable State")
            n201 = call "GLVT-Stepper-HWInteract.vi"("GLVT-Enable State"=w324) -> ()  [unwired: 10 in, 1 out]
            n202 = local write "GLVT-Motor State"(w324) -> ()
          }
          frame Error {
            n203 = call "Display Message to User5"("Message"="DAQ device not found.  Verify that the DAQ is off and safe.") -> ()  [unwired: 9 in, 2 out]
          }
        }
      }
    }
  }
  n204 = while "ANSI Loop" {
    shift-right: [w334] -> _
    shift-left: _ -> [w333]
    shift-right: [w337] -> w33
    shift-left: w1 -> [w332]
    shift-right: [w336] -> _
    shift-left: w36 -> [w338]
    tunnel: w31 -> [w331]
    shift-right: [w328] -> _
    shift-left: string[] [] -> [w329]
    i -> [w330]
    stop <- w335 stop-if-true
    # "ANSI Loop"
    n205 = call <vilib>:"Parse State Queue__JKI_lib_State_Machine.vi"("State Queue"=w338, "Error In (no error)"=w332) -> ("Remaining States"=w340:string, "Current State"=w327:string, "Arguments"=w339:string)  [unwired: 11 in]
    n206 = case shown="\"\", \"Idle\"" w327 {
      selector: w327 -> [_ _ w647 _ _ _ _ _ _ _ _ _ _ _ _ _ _ _ _ _ _ _ _]
      tunnel: w340 -> [w352 w646 w651 w669 w675 w682 w690 w705 w711 w715 w719 w725 w736 w762 w767 w777 w781 w804 w818 w833 w848 w853 w861]
      tunnel: w339 -> [_ _ _ _ _ _ _ _ _ _ _ w720 w730 _ _ _ _ _ _ _ _ _ _]
      tunnel: w333 -> [w350 w643 w649 w660 w672 w680 w687 _ w706 w712 w717 w723 w732 w759 w764 w774 w778 w788 w815 w824 w840 w851 w859]
      tunnel: [w349 w644 w653 w666 errorcluster {"status"=FALSE, "code"=0, "source"=""} ("error out") w676 w688 w702 w707 w713 w716 w721 w733 w760 w765 w775 w779 w783 w811 w825 w839 w850 w858] -> w337
      tunnel: w332 -> [w348 w644 w652 w666 w671 w677 w688 w702 w708 w713 w716 w722 w734 w760 w765 w775 w779 w790 w812 w826 w842 w850 w858]
      tunnel: [w351 w645 w650 w668 w674 w681 w689 w704 w710 w714 w718 w724 w735 w761 w766 w776 w780 w803 w817 w832 w847 w852 w860] -> w336
      tunnel: [_ _ _ _ _ w678 _ _ _ _ _ _ _ _ _ _ _ _ _ _ _ _ _] -> w335
      tunnel: [w347 w643 w649 w667 w672 w680 w687 w703 w706 w712 w717 w723 w732 w759 w764 w774 w778 w787 w814 w828 w841 w851 w859] -> w334
      tunnel: w331 -> [w346 _ _ _ _ _ _ w697 _ _ _ _ _ _ _ _ _ _ _ _ _ _ _]
      frame "", "Idle" {
        n207 = event shown="[18] \"Meter Select\": Value Change" {
          selector: _ -> [_ _ _ _ _ _ _ _ _ _ _ _ _ _ _ _ _ _ _ _ _ _ _ _ _ _ _ _ _]
          dyn-events: _ -> [_ _ _ _ _ _ _ _ _ _ _ _ _ _ _ _ _ _ _ _ _ _ _ _ _ _ _ _ _]
          timeout: 1000 -> [_ _ _ _ _ _ _ _ _ _ _ _ _ _ _ _ _ _ _ _ _ _ _ _ _ _ _ _ _]
          tunnel: w352 -> [w376 w398 w404 w410 w411 w421 w439 w445 w454 w463 w470 w490 w538 w542 w546 w548 w553 w558 w562 w565 w569 w573 w578 w582 w593 w609 w625 w634 w640]
          tunnel: [w361 w398 w404 w410 w411 w421 w439 w445 w454 w463 w470 w490 w538 w542 w546 w548 w553 w558 w562 w565 w569 w573 w578 w582 w593 w609 w625 w633 w639] -> w351
          tunnel: w350 -> [w360 w396 w402 w408 w412 w422 w440 w446 w455 w464 w472 w491 w539 w543 w547 w549 w554 w559 w563 w566 w570 w574 w579 w583 w594 w610 w626 w635 w641]
          tunnel: [w356 w397 w403 w409 w413 w423 w431 w443 w450 w459 w473 w487 w536 w540 w545 w550 w552 w557 w561 w567 w571 w575 w577 w581 w590 w606 w622 w636 w637] -> w349
          tunnel: w348 -> [w357 w397 w403 w409 w414 w424 w433 w447 w456 w466 w474 w488 w536 w540 w545 w550 w552 w557 w561 w567 w571 w575 w577 w581 w591 w608 w624 w636 w637]
          tunnel: [w360 w395 w401 w407 w412 w422 w440 w446 w455 w464 w471 w491 w539 w543 w547 w549 w554 w559 w563 w566 w570 w574 w579 w583 w594 w610 w626 w635 w641] -> w347
          tunnel: w346 -> [_ _ _ _ w415 w425 w432 w448 w457 w465 _ w486 _ _ _ _ _ _ _ _ _ _ _ _ w584 w600 w616 _ _]
          event Timeout {
            n208 = event-data() -> ()  [unwired: 1 in, 1 out]
            n209 = Unbundle By Name(w360) -> ("Start Data Save"=w358:bool)
            n210 = Or(x="Start ANSI 3", y="Start ANSI-S3") -> (x .or. y?=w355:bool)
            "ANSI 3" <- w355
            n211 = call <vilib>:"Add State(s) to Queue__jki_lib_state_machine.vi"("State(s) in Front (\"\")"="Check Exit\nUpdate Averages" ("State(s) in Front (\"\")"), "State(s) in (\"\")"=w376) -> ("States Out"=w374:string)  [unwired: 13 in]
            n212 = case shown="False" w358 {
              tunnel: ["" ("State(s) in Front (\"\")") "Save Data" ("State(s) in Front (\"\")")] -> w359
              tunnel: w357 -> [w377 w379]
              tunnel: [w377 w379] -> w356
              frame False {
              }
              frame True {
              }
            }
            n213 = case shown="True" w355 {
              tunnel: w374 -> [w389 w392]
              tunnel: [w389 w391] -> w373
              tunnel: "ANSI Average Bank 3" ("State(s) in Front (\"\")") -> [_ w390]
              frame False {
              }
              frame True {
                n214 = call <vilib>:"Add State(s) to Queue__jki_lib_state_machine.vi"("State(s) in Front (\"\")"=w390, "State(s) in (\"\")"=w392) -> ("States Out"=w391:string)  [unwired: 13 in]
              }
            }
            n215 = Or(x="Start ANSI 2", y="Start ANSI-S2") -> (x .or. y?=w353:bool)
            "ANSI 2" <- w353
            n216 = case shown="True" w353 {
              tunnel: w373 -> [w385 w388]
              tunnel: [w385 w387] -> w372
              tunnel: "ANSI Average Bank 2" ("State(s) in Front (\"\")") -> [_ w386]
              frame False {
              }
              frame True {
                n217 = call <vilib>:"Add State(s) to Queue__jki_lib_state_machine.vi"("State(s) in Front (\"\")"=w386, "State(s) in (\"\")"=w388) -> ("States Out"=w387:string)  [unwired: 13 in]
              }
            }
            n218 = Or(x="Start ANSI", y="Start ANSI-S1") -> (x .or. y?=w354:bool)
            "ANSI 1" <- w354
            n219 = case shown="False" w354 {
              tunnel: w372 -> [w381 w384]
              tunnel: [w381 w383] -> w362
              tunnel: "ANSI Average Bank 1" ("State(s) in Front (\"\")") -> [_ w382]
              frame False {
              }
              frame True {
                n220 = call <vilib>:"Add State(s) to Queue__jki_lib_state_machine.vi"("State(s) in Front (\"\")"=w382, "State(s) in (\"\")"=w384) -> ("States Out"=w383:string)  [unwired: 13 in]
              }
            }
            n221 = call <vilib>:"Add State(s) to Queue__jki_lib_state_machine.vi"("State(s) in Front (\"\")"=w359, "State(s) in (\"\")"=w362) -> ("States Out"=w361:string)  [unwired: 13 in]
          }
          event "Start ANSI": Value Change {
            n222 = event-data() -> ()  [unwired: 1 in, 6 out]
            n223 = local write "ANSI Display 1"("" ("ANSI Display 1")) -> ()
            n224 = Bundle By Name(cluster=w396, "Bank 1 Counter"=0) -> (w395:T29)
          }
          event "Start ANSI 2": Value Change {
            n225 = event-data() -> ()  [unwired: 1 in, 6 out]
            n226 = Bundle By Name(cluster=w402, "Bank 2 Counter"=0) -> (w401:T29)
            n227 = local write "ANSI Display 2"("" ("ANSI Display 2")) -> ()
          }
          event "Start ANSI 3": Value Change {
            n228 = event-data() -> ()  [unwired: 1 in, 6 out]
            n229 = local write "ANSI Display 3"("" ("ANSI Display 3")) -> ()
            n230 = Bundle By Name(cluster=w408, "Bank 3 Counter"=0) -> (w407:T29)
          }
          event "Change Gas Meter Bank1": Value Change {
            n231 = event-data() -> ()  [unwired: 1 in, 6 out]
            n232 = local read "Meter Select"() -> (w419:T4)
            n233 = call "RANGE Meter Bank Select.vi"("Error In"=w414, "Meter Data"=w415, "Meter Select"=w419) -> ("Error Out"=w417:errorcluster, "Unit ID"=w418:string, "VISA Refnum out"=w416:refnum<visa-resource-name>)  [unwired: 6 in]
            n234 = call "FMA1600A Create Custom Gas Mixture.vi"("Gas Type"="Gas Type", "Error In"=w417, "Unit ID"=w418, "VISA Refnum in"=w416) -> ("Error Out"=w413:errorcluster)  [unwired: 6 in, 1 out]
          }
          event "Change Gas Meter Bank 2": Value Change {
            n235 = event-data() -> ()  [unwired: 1 in, 6 out]
            n236 = local read "Meter Select 2"() -> (w428:T5)
            n237 = call "RANGE Meter Bank Select 2.vi"("Error In"=w424, "Meter Data"=w425, "Meter Select 2"=w428) -> ("Error Out"=w430:errorcluster, "Unit ID"=w427:string, "VISA Refnum out"=w429:refnum<visa-resource-name>)  [unwired: 6 in]
            n238 = call "FMA1600A Create Custom Gas Mixture.vi"("Gas Type"="Gas Type 2", "Error In"=w430, "Unit ID"=w427, "VISA Refnum in"=w429) -> ("Error Out"=w423:errorcluster)  [unwired: 6 in, 1 out]
          }
          event "Change Gas Meter Bank 3": Value Change {
            n239 = event-data() -> ()  [unwired: 1 in, 6 out]
            n240 = local read "Meter Select 3"() -> (w438:T6)
            n241 = call "RANGE Meter Bank Select 3.vi"("Error In"=w433, "Meter Data"=w432, "Meter Select Bank 3"=w438) -> ("Error Out"=w437:errorcluster, "Unit ID"=w434:string, "VISA Refnum out"=w435:refnum<visa-resource-name>)  [unwired: 6 in]
            n242 = call "FMA1600A Create Custom Gas Mixture.vi"("Gas Type"="Gas Type 3", "Error In"=w437, "Unit ID"=w434, "VISA Refnum in"=w435) -> ("Error Out"=w431:errorcluster)  [unwired: 6 in, 1 out]
          }
          event "Tare Meter Bank 1": Value Change {
            n243 = event-data() -> ()  [unwired: 1 in, 6 out]
            n244 = local read "Meter Select"() -> (w449:T4)
            n245 = call "RANGE Meter Bank Select.vi"("Error In"=w447, "Meter Data"=w448, "Meter Select"=w449) -> ("Error Out"=w444:errorcluster, "Unit ID"=w442:string, "VISA Refnum out"=w441:refnum<visa-resource-name>)  [unwired: 6 in]
            n246 = call "Tare Flow.vi"("Unit ID (A)"=w442, "error in"=w444, "VISA Session In"=w441) -> ("error out"=w443:errorcluster)  [unwired: 7 in, 1 out]
          }
          event "Tare Meter Bank 2": Value Change {
            n247 = event-data() -> ()  [unwired: 1 in, 6 out]
            n248 = local read "Meter Select 2"() -> (w458:T5)
            n249 = call "RANGE Meter Bank Select 2.vi"("Error In"=w456, "Meter Data"=w457, "Meter Select 2"=w458) -> ("Error Out"=w453:errorcluster, "Unit ID"=w451:string, "VISA Refnum out"=w452:refnum<visa-resource-name>)  [unwired: 6 in]
            n250 = call "Tare Flow.vi"("Unit ID (A)"=w451, "error in"=w453, "VISA Session In"=w452) -> ("error out"=w450:errorcluster)  [unwired: 7 in, 1 out]
          }
          event "Tare Meter Bank 3": Value Change {
            n251 = event-data() -> ()  [unwired: 1 in, 6 out]
            n252 = local read "Meter Select 3"() -> (w467:T6)
            n253 = call "RANGE Meter Bank Select 3.vi"("Error In"=w466, "Meter Data"=w465, "Meter Select Bank 3"=w467) -> ("Error Out"=w462:errorcluster, "Unit ID"=w461:string, "VISA Refnum out"=w460:refnum<visa-resource-name>)  [unwired: 6 in]
            n254 = call "Tare Flow.vi"("Unit ID (A)"=w461, "error in"=w462, "VISA Session In"=w460) -> ("error out"=w459:errorcluster)  [unwired: 7 in, 1 out]
          }
          event "Record": Value Change {
            n255 = event-data() -> ("NewVal"=w469:bool)  [unwired: 1 in, 5 out]
            n256 = case shown="True" w469 {
              tunnel: w474 -> [w476 w483]
              tunnel: [w476 w482] -> w473
              tunnel: [path "" ("Path") w481] -> w468
              frame False {
              }
              frame True {
                n257 = local read "Meter 3/4"() -> (w477:string)
                n258 = local read "Meter 1/2"() -> (w478:string)
                n259 = local read "All Meter Data"() -> (w480:T13)
                n260 = local read "Meter 5/6"() -> (w479:string)
                n261 = call "RANGE Create File.vi"("Meter 3/4"=w477, "Meter 5/6"=w479, "Meter 1/2"=w478, "Error In"=w483, "All Meter Data"=w480) -> ("Error Out"=w482:errorcluster, "Path"=w481:path)  [unwired: 5 in]
              }
            }
            n262 = Bundle By Name(cluster=w472, "Start Data Save"=w469, "File Path"=w468) -> (w471:T29)
            n263 = local write "File Path"(w468) -> ()
          }
          event "Manual Commands": Value Change {
            n264 = event-data() -> ()  [unwired: 1 in, 6 out]
            n265 = case shown="\"F\"" "Unit ID (A-F)" {
              tunnel: "FMA1600A Commands" -> [_ w499 w506 w509 w518 w523 w530]
              tunnel: w488 -> [w493 w496 w505 w510 w515 w527 w534]
              tunnel: [w493 w495 w504 w511 w520 w526 w533] -> w487
              tunnel: "Unit ID (A-F)" -> [_ w498 w501 w508 w517 w522 w531]
              tunnel: w486 -> [_ w500 w507 w514 w521 w528 w535]
              tunnel: ["" ("Raw FMA1600A Data") w494 w502 w512 w519 w525 w532] -> w484
              frame Default {
              }
              frame "A" {
                n266 = Unbundle By Name(w500) -> ("Meter 1.Meter Visa"=w497:refnum<visa-resource-name>)
                n267 = call "FMA1600A General Send Receive.vi"("error in (no error)"=w496, "Unit ID in"=w498, "FMA1600A Commands"=w499, "VISA Refnum in"=w497) -> ("error out"=w495:errorcluster, "Data Stream"=w494:string)  [unwired: 4 in, 2 out]
              }
              frame "B" {
                n268 = Unbundle By Name(w507) -> ("Meter 2.Meter Visa"=w503:refnum<visa-resource-name>)
                n269 = call "FMA1600A General Send Receive.vi"("error in (no error)"=w505, "Unit ID in"=w501, "FMA1600A Commands"=w506, "VISA Refnum in"=w503) -> ("error out"=w504:errorcluster, "Data Stream"=w502:string)  [unwired: 4 in, 2 out]
              }
              frame "C" {
                n270 = Unbundle By Name(w514) -> ("Meter 3.Meter Visa"=w513:refnum<visa-resource-name>)
                n271 = call "FMA1600A General Send Receive.vi"("error in (no error)"=w510, "Unit ID in"=w508, "FMA1600A Commands"=w509, "VISA Refnum in"=w513) -> ("error out"=w511:errorcluster, "Data Stream"=w512:string)  [unwired: 4 in, 2 out]
              }
              frame "D" {
                n272 = Unbundle By Name(w521) -> ("Meter 4.Meter Visa"=w516:refnum<visa-resource-name>)
                n273 = call "FMA1600A General Send Receive.vi"("error in (no error)"=w515, "Unit ID in"=w517, "FMA1600A Commands"=w518, "VISA Refnum in"=w516) -> ("error out"=w520:errorcluster, "Data Stream"=w519:string)  [unwired: 4 in, 2 out]
              }
              frame "E" {
                n274 = Unbundle By Name(w528) -> ("Meter 5.Meter Visa"=w524:refnum<visa-resource-name>)
                n275 = call "FMA1600A General Send Receive.vi"("error in (no error)"=w527, "Unit ID in"=w522, "FMA1600A Commands"=w523, "VISA Refnum in"=w524) -> ("error out"=w526:errorcluster, "Data Stream"=w525:string)  [unwired: 4 in, 2 out]
              }
              frame "F" {
                n276 = Unbundle By Name(w535) -> ("Meter 6.Meter Visa"=w529:refnum<visa-resource-name>)
                n277 = call "FMA1600A General Send Receive.vi"("error in (no error)"=w534, "Unit ID in"=w531, "FMA1600A Commands"=w530, "VISA Refnum in"=w529) -> ("error out"=w533:errorcluster, "Data Stream"=w532:string)  [unwired: 4 in, 2 out]
              }
            }
            "Raw FMA1600A Data" <- w484
          }
          event "HeatingValueS1": Value Change {
            n278 = event-data() -> ()  [unwired: 1 in, 6 out]
            n279 = local read "HeatingValueS1"() -> (w537:dbl)
            n280 = local write "HeatingValue Meter 1/2"(w537) -> ()
          }
          event "HeatingValueS2": Value Change {
            n281 = event-data() -> ()  [unwired: 1 in, 6 out]
            n282 = local read "HeatingValueS2"() -> (w541:dbl)
            n283 = local write "HeatingValue Meter 3/4"(w541) -> ()
          }
          event "HeatingValueS3": Value Change {
            n284 = event-data() -> ()  [unwired: 1 in, 6 out]
            n285 = local read "HeatingValueS3"() -> (w544:dbl)
            n286 = local write "HeatingValue Meter 5/6"(w544) -> ()
          }
          event "HeatingValue Meter 1/2": Value Change {
            n287 = event-data() -> ()  [unwired: 1 in, 6 out]
            n288 = local read "HeatingValue Meter 1/2"() -> (w551:dbl)
            n289 = local write "HeatingValueS1"(w551) -> ()
          }
          event "HeatingValue Meter 3/4": Value Change {
            n290 = event-data() -> ()  [unwired: 1 in, 6 out]
            n291 = local read "HeatingValue Meter 3/4"() -> (w555:dbl)
            n292 = local write "HeatingValueS2"(w555) -> ()
          }
          event "HeatingValue Meter 5/6": Value Change {
            n293 = event-data() -> ()  [unwired: 1 in, 6 out]
            n294 = local read "HeatingValue Meter 5/6"() -> (w556:dbl)
            n295 = local write "HeatingValueS3"(w556) -> ()
          }
          event Value Change {
            n296 = event-data() -> ()  [unwired: 1 in, 6 out]
            n297 = local read "Meter Select"() -> (w560:T4)
            n298 = local write "Meter Select 1/2"(w560) -> ()
          }
          event Value Change {
            n299 = event-data() -> ()  [unwired: 1 in, 6 out]
            n300 = local read "Meter Select 2"() -> (w564:T5)
            n301 = local write "Meter Select 3/4"(w564) -> ()
          }
          event Value Change {
            n302 = event-data() -> ()  [unwired: 1 in, 6 out]
            n303 = local read "Meter Select 3"() -> (w568:T6)
            n304 = local write "Meter Select 5/6"(w568) -> ()
          }
          event Value Change {
            n305 = event-data() -> ()  [unwired: 1 in, 6 out]
            n306 = local write "Meter Select"("Meter Select 1/2") -> ()
          }
          event Value Change {
            n307 = event-data() -> ()  [unwired: 1 in, 6 out]
            n308 = local write "Meter Select 2"("Meter Select 3/4") -> ()
          }
          event Value Change {
            n309 = event-data() -> ()  [unwired: 1 in, 6 out]
            n310 = local write "Meter Select 3"("Meter Select 5/6") -> ()
          }
          event "Reset Totalizer Bank 1": Value Change {
            n311 = event-data() -> ()  [unwired: 1 in, 6 out]
            n312 = local read "Meter Select"() -> (w586:T4)
            n313 = call "RANGE Meter Bank Select.vi"("Error In"=w591, "Meter Data"=w584, "Meter Select"=w586) -> ("Error Out"=w592:errorcluster, "Unit ID"=w585:string, "VISA Refnum out"=w589:refnum<visa-resource-name>)  [unwired: 6 in]
            n314 = Equal?(x=refnum<visa-resource-name> refnum, y=w589) -> (x = y?=w587:bool)
            n315 = case shown="False" w587 {
              tunnel: w592 -> [w598 w599]
              tunnel: [w597 w599] -> w590
              tunnel: w589 -> [w596 _]
              tunnel: w585 -> [w595 _]
              frame False {
                n316 = call "Reset Totalizer.vi"("Unit ID (A)"=w595, "error in"=w598, "VISA Session In"=w596) -> ("error out"=w597:errorcluster)  [unwired: 6 in, 2 out]
              }
              frame True {
              }
            }
          }
          event "Reset Totalizer Bank 2": Value Change {
            n317 = event-data() -> ()  [unwired: 1 in, 6 out]
            n318 = local read "Meter Select 2"() -> (w602:T5)
            n319 = call "RANGE Meter Bank Select 2.vi"("Error In"=w608, "Meter Data"=w600, "Meter Select 2"=w602) -> ("Error Out"=w607:errorcluster, "Unit ID"=w601:string, "VISA Refnum out"=w605:refnum<visa-resource-name>)  [unwired: 6 in]
            n320 = Equal?(x=refnum<visa-resource-name> refnum, y=w605) -> (x = y?=w603:bool)
            n321 = case shown="False" w603 {
              tunnel: w607 -> [w614 w615]
              tunnel: [w613 w615] -> w606
              tunnel: w605 -> [w612 _]
              tunnel: w601 -> [w611 _]
              frame False {
                n322 = call "Reset Totalizer.vi"("Unit ID (A)"=w611, "error in"=w614, "VISA Session In"=w612) -> ("error out"=w613:errorcluster)  [unwired: 6 in, 2 out]
              }
              frame True {
              }
            }
          }
          event "Reset Totalizer Bank 3": Value Change {
            n323 = event-data() -> ()  [unwired: 1 in, 6 out]
            n324 = local read "Meter Select 3"() -> (w618:T6)
            n325 = call "RANGE Meter Bank Select 3.vi"("Error In"=w624, "Meter Data"=w616, "Meter Select Bank 3"=w618) -> ("Error Out"=w623:errorcluster, "Unit ID"=w617:string, "VISA Refnum out"=w621:refnum<visa-resource-name>)  [unwired: 6 in]
            n326 = Equal?(x=refnum<visa-resource-name> refnum, y=w621) -> (x = y?=w619:bool)
            n327 = case shown="False" w619 {
              tunnel: w623 -> [w630 w631]
              tunnel: w621 -> [w628 _]
              tunnel: [w629 w631] -> w622
              tunnel: w617 -> [w627 _]
              frame False {
                n328 = call "Reset Totalizer.vi"("Unit ID (A)"=w627, "error in"=w630, "VISA Session In"=w628) -> ("error out"=w629:errorcluster)  [unwired: 6 in, 2 out]
              }
              frame True {
              }
            }
          }
          event "Exit Button": Value Change {
            n329 = event-data() -> ()  [unwired: 1 in, 6 out]
            n330 = call <vilib>:"Add State(s) to Queue__jki_lib_state_machine.vi"("State(s) in Front (\"\")"="Macro: Exit" ("State(s) in Front (\"\")"), "State(s) in (\"\")"=w634) -> ("States Out"=w633:string)  [unwired: 13 in]
          }
          event Panel Close? {
            n331 = event-data() -> ()  [unwired: 1 in, 4 out]
            n332 = call <vilib>:"Add State(s) to Queue__jki_lib_state_machine.vi"("State(s) in Front (\"\")"="Macro: Exit" ("State(s) in Front (\"\")"), "State(s) in (\"\")"=w640) -> ("States Out"=w639:string)  [unwired: 13 in]
            n333 = event-data("Discard?"=TRUE) -> ()  [unwired: 1 in, 1 out]
          }
        }
      }
      frame "---------- Core ----------" {
        # "Do not put any code in this frame.\n(it is a separator no-op)"
        n334 = call <vilib>:"Add State(s) to Queue__jki_lib_state_machine.vi"("State(s) in (\"\")"=w646) -> ("States Out"=w645:string)  [unwired: 14 in]
      }
      frame Default {
        w656 = 42 items=["No error", "Argument error", "Memory is full", "Out of zone", "End of file", "File already open", "Generic file I/O error", "File not found", "File permission error", "Disk is full", "Duplicate path", "Too many files open", "System feature not enabled", "Resource file not found", "Cannot add resource", "Resource not found", "Image not found", "Image memory error", "Pen does not exist", "Config type invalid", "Config token not found", "Config parse error", "Config memory error", "Bad external code format", "Bad external code offset", "External code not present", "Null window", "Destroy window error", "Null menu", "Print aborted", "Bad print record", "Print driver error", "Windows error during printing", "Memory error during printing", "Print dialog error", "Generic print error", "Invalid device refnum", "Device not found", "Device parameter error", "Device unit error", "Cannot open device", "Device call aborted", "Generic error", "Cancelled by user", "Object ID too low", "Object ID too high", "Object not in heap", "Unknown heap", "Unknown object (invalid DefProc)", "Unknown object (DefProc not in table)", "Message out of range", "Invalid (null) method", "Unknown message", "Manager call not supported", "Bad address", "Network operation in progress", "Network operation timed out", "Connection is busy", "Network attribute not supported", "Network error", "Address in use", "System out of memory", "Connection aborted", "Connection refused", "Not connected", "Already connected", "Connection closed", "Initialization error (interapplication manager)", "Bad occurrence", "Wait on unbound occurrence handler", "Occurrence queue overflow", "Datalog type conflict", "Unused", "Unrecognized type (interapplication manager)", "Memory corrupt", "Failed to make temporary DLL", "Old CIN version", "Drag socket not found", "Failed to load drop-object", "Failed to register OLE object", "Failed to release OLE object", "Format specifier type mismatch", "Unknown format specifier", "Too few format specifiers", "Too many format specifiers", "Scan failed", "Newer CIN version", "Error converting to variant", "Runtime menu error", "Password tampered", "Variant attribute not found", "Incompatible variant data type", "Event data is not available", "Event Store is not present", "Occurrence is not found", "Event Queue is not created", "Event info is not available", "Refnum passed is NULL", "Error retrieving Class GUID", "Error retrieving CoClass GUID", "Error retrieving TypeLib GUID.", "Bad built application magic bytes.", "Specific driver is different from the specific driver associated with the Logical Name.", "There is no session opened to the class driver.", "Max Error", "MAX - Error with config objects", "MAX - Error loading configuration", "MAX - Group not supported"]
        # "Current State"
        # "Do not delete, rename, or modify this frame.\n(this is used to capture unhandled states and typos)"
        # "Handle mistyped state name (developer tool)"
        n335 = Format Into String(format string="Software Exception: Unhandled State \"%s\"." ("message"), error in=w652, w647) -> (resulting string=w655:string, error out=w654:errorcluster)  [unwired: 1 in]
        n336 = call <vilib>:"Error Cluster From Error Code.vi"("show call chain? (False)"=TRUE, "error in (no error)"=w654, "error message (\"\")"=w655, "error code (0)"=w656) -> ("error out"=w653:errorcluster)  [unwired: 5 in]
        n337 = call <vilib>:"Add State(s) to Queue__jki_lib_state_machine.vi"("State(s) in (\"\")"=w651) -> ("States Out"=w650:string)  [unwired: 14 in]
      }
      frame "Initialize Core Data" {
        # "Do not delete, rename, or modify this frame.\n(this is used to determine panel behavior on exit)"
        # "originally closed?"
        # "exe?"
        # "If panel starts closed or is an EXE, then close it when we exit"
        n338 = property class="App"() -> ("App.Kind"=w664:T26)  [unwired: 2 in, 2 out]
        n339 = property class="VI"() -> ("Front Panel.Open"=w665:bool)  [unwired: 2 in, 2 out]
        n340 = control-ref of="Current VI Reference"() -> (w658:refnum<vi>)
        n341 = Not(x=w665) -> (.not. x?=w662:bool)
        n342 = Equal?(x=w664, y=T26."Run Time System" ("Application:Kind")) -> (x = y?=w661:bool)
        n343 = Or(x=w662, y=w661) -> (x .or. y?=w659:bool)
        n344 = Bundle By Name(cluster=w660, "Core.Current VI Reference"=w658, "Core.Close Panel on Exit?"=w659) -> (w667:T29)
        n345 = call <vilib>:"Add State(s) to Queue__jki_lib_state_machine.vi"("State(s) in (\"\")"=w669) -> ("States Out"=w668:string)  [unwired: 14 in]
      }
      frame "Error Handler" {
        # "Unhandled Error -- Display it"
        # "Handle any errors here.\nYou can also output any states to clean-up after errors occur"
        # "Clear error"
        n346 = call <vilib>:"General Error Handler.vi"("error in (no error)"=w671) -> ()  [unwired: 10 in, 5 out]
        n347 = call <vilib>:"Add State(s) to Queue__jki_lib_state_machine.vi"("State(s) in Front (\"\")"="/* Post Error States", "State(s) in (\"\")"=w675) -> ("States Out"=w674:string)  [unwired: 13 in]
      }
      frame "Exit" {
        w678 = TRUE
        # "Do not put any code in this frame.\n(No errors that occur here will be handled.)"
        n348 = for {
          N: 6 -> [_]
          tunnel: w678 -> [w684]
          shift-right: [w683] -> w676
          shift-left: w677 -> [w683]
          n349 = call "UTILITY Boolean Notifier.vi"("Status"=UTILITY_Notifier."Set", "Set Status"=w684, "name (unnamed)"="Exit") -> ()  [unwired: 7 in, 2 out]
        }
        n350 = call <vilib>:"Add State(s) to Queue__jki_lib_state_machine.vi"("State(s) in (\"\")"=w682) -> ("States Out"=w681:string)  [unwired: 14 in]
      }
      frame "---------- Data ----------" {
        # "Do not put any code in this frame.\n(It is a separator no-op. You can make a copy of this frame to create a new Data frame)"
        n351 = call <vilib>:"Add State(s) to Queue__jki_lib_state_machine.vi"("State(s) in (\"\")"=w690) -> ("States Out"=w689:string)  [unwired: 14 in]
      }
      frame "Data: Initialize" {
        w694 = 0.0  # Elapsed Time DAQ
        w696 = FALSE  # Start Data Save
        w698 = 0  # Bank 3 Counter
        w699 = 0  # Bank 2 Counter
        w700 = 0  # Bank 1 Counter
        w701 = T30 {"Current VI Reference"=refnum, "Close Panel on Exit?"=FALSE}  # Core
        # "These transfer data to the main heating value control"
        # "Initialize the shift-register data, here.\n(data names are defined by what you wire into the bundle function)"
        n352 = local read "HeatingValueS1"() -> (w693:dbl)
        n353 = local read "HeatingValueS2"() -> (w692:dbl)
        n354 = local read "HeatingValueS3"() -> (w691:dbl)
        n355 = local write "HeatingValue Meter 1/2"(w693) -> ()
        n356 = local write "HeatingValue Meter 3/4"(w692) -> ()
        n357 = local write "HeatingValue Meter 5/6"(w691) -> ()
        n358 = Bundle("Core"=w701, "Bank 1 Counter"=w700, "Bank 2 Counter"=w699, "Bank 3 Counter"=w698, "Meter Data"=w697, "File Path"="File Path", "Start Data Save"=w696, "Elapsed Time DAQ"=w694) -> (w703:T29)  [unwired: 1 in]
        n359 = call <vilib>:"Add State(s) to Queue__jki_lib_state_machine.vi"("State(s) in (\"\")"=w705) -> ("States Out"=w704:string)  [unwired: 14 in]
      }
      frame "Data: Cleanup" {
        # "Cleanup any data and references, here.\n(this is called automatically, by the Macro: Exit)"
        n360 = Unbundle By Name(w706) -> ("Core.Current VI Reference"=w709:refnum<vi>)
        n361 = Close Reference(reference=w709, error in (no error)=w708) -> (error out=w707:errorcluster)
        n362 = call <vilib>:"Add State(s) to Queue__jki_lib_state_machine.vi"("State(s) in (\"\")"=w711) -> ("States Out"=w710:string)  [unwired: 14 in]
      }
      frame "---------- UI ----------" {
        # "Do not put any code in this frame.\n(It is a separator no-op. You can make a copy of this frame to create a new UI frame)"
        n363 = call <vilib>:"Add State(s) to Queue__jki_lib_state_machine.vi"("State(s) in (\"\")"=w715) -> ("States Out"=w714:string)  [unwired: 14 in]
      }
      frame "UI: Initialize" {
        # "Initialize the User Interface, here.\n(this is called automatically, by the Macro: Init)"
        n364 = call <vilib>:"Add State(s) to Queue__jki_lib_state_machine.vi"("State(s) in (\"\")"=w719) -> ("States Out"=w718:string)  [unwired: 14 in]
      }
      frame "UI: Cursor Set" {
        # "Argument"
        # "Set and Unset Cursor Busy.\n(Usage: \"UI: Cursor Set >> Busy|Idle\")"
        n365 = case shown="\"Idle\", Default" w720 {
          tunnel: w722 -> [w727 w729]
          tunnel: [w726 w728] -> w721
          frame "Idle", Default {
            n366 = call <vilib>:"Unset Busy.vi"("error in (no error)"=w727) -> ("error out"=w726:errorcluster)  [unwired: 10 in]
          }
          frame "Busy" {
            n367 = call <vilib>:"Set Busy.vi"("error in (no error)"=w729) -> ("error out"=w728:errorcluster)  [unwired: 9 in, 1 out]
          }
        }
        n368 = call <vilib>:"Add State(s) to Queue__jki_lib_state_machine.vi"("State(s) in (\"\")"=w725) -> ("States Out"=w724:string)  [unwired: 14 in]
      }
      frame "UI: Front Panel State" {
        # "Argument"
        # "Set Front Panel Open or Closed\n(Usage: \"UI: Front Panel State >> Open|Close\")"
        n369 = Unbundle By Name(w732) -> ("Core.Current VI Reference"=w731:refnum<vi>)
        n370 = case shown="\"Open\", Default" w730 {
          tunnel: w734 -> [w740 w753]
          tunnel: [w742 w754] -> w733
          tunnel: w731 -> [w741 w751]
          frame "Open", Default {
            n371 = property class="VI"(reference=w741, error in=w740) -> (reference out=w738:refnum<vi>, error out=w739:errorcluster, "Front Panel.Open"=w737:bool)
            n372 = case shown="True" w737 {
              tunnel: [w745 w748] -> w742
              tunnel: w739 -> [w744 w748]
              tunnel: w738 -> [w743 _]
              frame False {
                n373 = invoke class="VI" method="FP.Open"(reference=w743, error in=w744, "Activate"=TRUE, "State"=T27."Standard") -> (error out=w745:errorcluster)  [unwired: 1 in, 4 out]
              }
              frame True {
              }
            }
          }
          frame "Close" {
            n374 = property class="VI"(reference=w751, error in=w753) -> (reference out=w750:refnum<vi>, error out=w752:errorcluster, "Front Panel.Open"=w749:bool)
            n375 = case shown="True" w749 {
              tunnel: [w755 w758] -> w754
              tunnel: w752 -> [w755 w757]
              tunnel: w750 -> [_ w756]
              frame False {
              }
              frame True {
                n376 = invoke class="VI" method="FP.Close"(reference=w756, error in=w757) -> (error out=w758:errorcluster)  [unwired: 1 in, 2 out]
              }
            }
          }
        }
        n377 = call <vilib>:"Add State(s) to Queue__jki_lib_state_machine.vi"("State(s) in (\"\")"=w736) -> ("States Out"=w735:string)  [unwired: 14 in]
      }
      frame "---------- Macro ----------" {
        # "Do not put any code in this frame.\n(It is a separator no-op. You can make a copy of this frame to create a new Macro frame)"
        n378 = call <vilib>:"Add State(s) to Queue__jki_lib_state_machine.vi"("State(s) in (\"\")"=w762) -> ("States Out"=w761:string)  [unwired: 14 in]
      }
      frame "Macro: Initialize" {
        w763 = "Data: Initialize\nInitialize Core Data\nUI: Initialize\nUI: Front Panel State >> Open"  # Data: Initialize Initialize Core Data UI: Initialize UI: Front Panel State >> Open
        # "Initialization Macro\n(This is called once, when the VI starts)"
        n379 = call <vilib>:"Add State(s) to Queue__jki_lib_state_machine.vi"("State(s) in Front (\"\")"=w763, "State(s) in (\"\")"=w767) -> ("States Out"=w766:string)  [unwired: 13 in]
      }
      frame "Macro: Exit" {
        # "Exit Macro\n(This is called once, when the VI exits)"
        n380 = Unbundle By Name(w774) -> ("Core.Close Panel on Exit?"=w773:bool)
        n381 = Select(t="UI: Front Panel State >> Close", s=w773, f="") -> (s? t:f=w770:string)
        n382 = call <vilib>:"Add State(s) to Queue__jki_lib_state_machine.vi"("State(s) in (\"\")"=w770, "State(s) at Back (\"\")"="Data: Cleanup\nExit") -> ("States Out"=w768:string)  [unwired: 13 in]
        n383 = call <vilib>:"Add State(s) to Queue__jki_lib_state_machine.vi"("State(s) in Front (\"\")"=w768, "State(s) in (\"\")"=w777) -> ("States Out"=w776:string)  [unwired: 13 in]
      }
      frame "---------- New Category ----------" {
        # "Template Separator\n(You can make a copy of, or modify, this frame)"
        n384 = call <vilib>:"Add State(s) to Queue__jki_lib_state_machine.vi"("State(s) in (\"\")"=w781) -> ("States Out"=w780:string)  [unwired: 14 in]
      }
      frame "Update Averages" {
        n385 = local read "All Meter Data"() -> (w794:T13)
        n386 = Unbundle By Name(w788) -> ("Meter Data"=w789:T13)
        n387 = Unbundle By Name(w794) -> ("Meter Bank 1.Flow Rate (BTU/HR)"=w793:dbl, "Meter Bank 2.Flow Rate (BTU/HR)"=w792:dbl, "Meter Bank 3.Flow Rate (BTU/HR)"=w791:dbl)
        n388 = Bundle By Name(cluster=w789, "Meter Bank 1.Flow Rate (BTU/HR)"=w793, "Meter Bank 2.Flow Rate (BTU/HR)"=w792, "Meter Bank 3.Flow Rate (BTU/HR)"=w791) -> (w795:T13)
        n389 = call <vilib>:"Add State(s) to Queue__jki_lib_state_machine.vi"("State(s) in (\"\")"=w804) -> ("States Out"=w803:string)  [unwired: 14 in]
        n390 = call "RANGE Average Flow Rates.vi"("All Meter Data"=w795, "Error In"=w790, "Meter Number"=Range_Meter_Bank."Meter Bank 1") -> ("All Meter Data Out"=w800:T13, "Error Out"=w801:errorcluster)  [unwired: 15 in]
        n391 = call "RANGE Average Flow Rates.vi"("All Meter Data"=w800, "Error In"=w801, "Meter Number"=Range_Meter_Bank."Meter Bank 2") -> ("All Meter Data Out"=w799:T13, "Error Out"=w802:errorcluster)  [unwired: 15 in]
        n392 = call "RANGE Average Flow Rates.vi"("All Meter Data"=w799, "Error In"=w802, "Meter Number"=Range_Meter_Bank."Meter Bank 3") -> ("All Meter Data Out"=w786:T13, "Error Out"=w784:errorcluster)  [unwired: 15 in]
        "Average Updates" <- w786
        n393 = call "UTILITY Elapsed Time.vi"("error in (no error)"=w784) -> ("error out"=w783:errorcluster, "Main Loop Rate"=→"Main Loop Rate":dbl, "Elapsed Time"=w782:dbl)  [unwired: 6 in, 2 out]
        "Elapsed Time" <- w782
        n394 = Bundle By Name(cluster=w788, "Meter Data"=w786, "Elapsed Time DAQ"=w782) -> (w787:T29)
      }
      frame "ANSI Average Bank 1" {
        n395 = local read "All Meter Data"() -> (w816:T13)
        n396 = Unbundle By Name(w815) -> ("Bank 1 Counter"=w813:i32)
        n397 = call "RANGE ANSI Calculator.vi"("Meter Number"=Range_Meter_Bank."Meter Bank 1", "Error In"=w812, "All Meter Data"=w816, "Bank Counter"=w813) -> ("Error Out"=w811:errorcluster, "Count Down Timer"=w808:i32, "ANSI Average (BTU/HR)"=w806:dbl, "Bank Counter"=w807:i32, "Greater than 310 sec"=w810:bool)  [unwired: 3 in]
        "ANSI Average (BTU/hr)-Meter 1/2" <- w806
        n398 = case shown="True" w810 {
          frame False {
          }
          frame True {
            w819 = FALSE ("Start ANSI")
            n399 = local write "Start ANSI-S1"(w819) -> ()
            n400 = local write "Start ANSI"(w819) -> ()
          }
        }
        n401 = call "RANGE ANSI Message.vi"("Bank Counter"=w807, "Count Down Timer"=w808) -> ("ANSI Display 3"=→"ANSI Display 1" →"ANSI Display S1":string)  [unwired: 9 in]
        n402 = Bundle By Name(cluster=w815, "Bank 1 Counter"=w807) -> (w814:T29)
        n403 = local write "ANSI Average (BTU/hr)"(w806) -> ()
        n404 = call <vilib>:"Add State(s) to Queue__jki_lib_state_machine.vi"("State(s) in (\"\")"=w818) -> ("States Out"=w817:string)  [unwired: 14 in]
      }
      frame "ANSI Average Bank 2" {
        n405 = Unbundle By Name(w824) -> ("Bank 2 Counter"=w829:i32)
        n406 = local read "All Meter Data"() -> (w830:T13)
        n407 = call "RANGE ANSI Calculator.vi"("Meter Number"=Range_Meter_Bank."Meter Bank 2", "Error In"=w826, "All Meter Data"=w830, "Bank Counter"=w829) -> ("Error Out"=w825:errorcluster, "Count Down Timer"=w823:i32, "ANSI Average (BTU/HR)"=w821:dbl, "Bank Counter"=w822:i32, "Greater than 310 sec"=w831:bool)  [unwired: 3 in]
        "ANSI Average (BTU/hr)-Meter 3/4" <- w821
        n408 = case shown="False" w831 {
          frame False {
          }
          frame True {
            w834 = FALSE ("Start ANSI")
            n409 = local write "Start ANSI 2"(w834) -> ()
            n410 = local write "Start ANSI-S2"(w834) -> ()
          }
        }
        n411 = call "RANGE ANSI Message.vi"("Bank Counter"=w822, "Count Down Timer"=w823) -> ("ANSI Display 3"=→"ANSI Display 2" →"ANSI Display S2":string)  [unwired: 9 in]
        n412 = local write "ANSI Average (BTU/hr) 2"(w821) -> ()
        n413 = Bundle By Name(cluster=w824, "Bank 2 Counter"=w822) -> (w828:T29)
        n414 = call <vilib>:"Add State(s) to Queue__jki_lib_state_machine.vi"("State(s) in (\"\")"=w833) -> ("States Out"=w832:string)  [unwired: 14 in]
      }
      frame "ANSI Average Bank 3" {
        n415 = Unbundle By Name(w840) -> ("Bank 3 Counter"=w844:i32)
        n416 = local read "All Meter Data"() -> (w845:T13)
        n417 = call "RANGE ANSI Calculator.vi"("Meter Number"=Range_Meter_Bank."Meter Bank 3", "Error In"=w842, "All Meter Data"=w845, "Bank Counter"=w844) -> ("Error Out"=w839:errorcluster, "Count Down Timer"=w838:i32, "ANSI Average (BTU/HR)"=w836:dbl, "Bank Counter"=w837:i32, "Greater than 310 sec"=w846:bool)  [unwired: 3 in]
        "ANSI Average (BTU/hr)-Meter 5/6" <- w836
        n418 = case shown="True" w846 {
          frame False {
          }
          frame True {
            w849 = FALSE ("Start ANSI")
            n419 = local write "Start ANSI 3"(w849) -> ()
            n420 = local write "Start ANSI-S3"(w849) -> ()
          }
        }
        n421 = call "RANGE ANSI Message.vi"("Bank Counter"=w837, "Count Down Timer"=w838) -> ("ANSI Display 3"=→"ANSI Display 3" →"ANSI Display S3":string)  [unwired: 9 in]
        n422 = local write "ANSI Average (BTU/hr) 3"(w836) -> ()
        n423 = Bundle By Name(cluster=w840, "Bank 3 Counter"=w837) -> (w841:T29)
        n424 = call <vilib>:"Add State(s) to Queue__jki_lib_state_machine.vi"("State(s) in (\"\")"=w848) -> ("States Out"=w847:string)  [unwired: 14 in]
      }
      frame "Save Data" {
        n425 = call <vilib>:"Add State(s) to Queue__jki_lib_state_machine.vi"("State(s) in (\"\")"=w853) -> ("States Out"=w852:string)  [unwired: 14 in]
      }
      frame "Check Exit" {
        n426 = call "UTILITY Boolean Notifier.vi"("Status"=UTILITY_Notifier."Read", "name (unnamed)"="Exit") -> ("latest READ notification"=w855:bool)  [unwired: 8 in, 1 out]
        n427 = case shown="True" w855 {
          tunnel: ["" "Macro: Exit"] -> w854
          frame False {
          }
          frame True {
          }
        }
        n428 = call <vilib>:"Add State(s) to Queue__jki_lib_state_machine.vi"("State(s) in Front (\"\")"=w854, "State(s) in (\"\")"=w861) -> ("States Out"=w860:string)  [unwired: 13 in]
      }
    }
    n429 = case shown="False" "Debug" {
      tunnel: w329 -> [w341 w344]
      tunnel: [w341 w343] -> w328
      tunnel: w327 -> [_ w342]
      frame False {
      }
      frame True {
        n430 = Build Array (concatenate)(w344, w342) -> (w343:string[])
        "Debug Array" <- w343
      }
    }
    "ANSI Loop" <- w330
  }
  n431 = while {
    tunnel: w1 -> [w865]
    tunnel: [w865] -> w22
    i -> [w866]
    stop <- w867 stop-if-true
    n432 = event shown="[1] \"Meter 1/2\": Value Change" {
      selector: _ -> [_ _ _ _]
      dyn-events: _ -> [_ _ _ _]
      timeout: 200 -> [_ _ _ _]
      event Timeout {
        n433 = event-data() -> ()  [unwired: 1 in, 3 out]
      }
      event "Meter 1/2": Value Change {
        n434 = event-data() -> ("NewVal"=w870:string)  [unwired: 1 in, 5 out]
        n435 = local read "Meter Select"() -> (w871:T4)
        n436 = case shown="Default" w871 {
          tunnel: w870 -> [_ w878]
          frame Default {
          }
          frame "Auto" {
            n437 = local read "All Meter Data"() -> (w877:T13)
            n438 = Unbundle By Name(w877) -> ("Use Auto Switching"=w873:bool, "Meter Bank 1.Panel Data.Mass Flow"=w875:dbl)
            n439 = Greater Than 0?(x=w875) -> (x > 0?=w874:bool)
            n440 = And(x=w873, y=w874) -> (x .and. y?=w872:bool)
            n441 = case shown="True" w872 {
              tunnel: [TRUE w883] -> w876
              frame False {
              }
              frame True {
                n442 = local read "Tab Control 2"() -> (w881:T2)
                n443 = Equal?(x=w881, y=RANGE_Tab_Control_2."All Stations" ("Tab Control 2")) -> (x = y?=w885:bool)
                n444 = Equal?(x=w881, y=RANGE_Tab_Control_2."Custom Gases") -> (x = y?=w884:bool)
                n445 = Equal?(x=w881, y=RANGE_Tab_Control_2."Gas Valve Flow Test") -> (x = y?=w880:bool)
                n446 = Compound Arithmetic op=OR(w885, w884, w880) -> (w883:bool)
              }
            }
            n447 = case shown="False" w876 {
              tunnel: w878 -> [w888 _]
              frame False {
                n448 = case shown="\"1\", \"2\"" w888 {
                  frame Default {
                  }
                  frame "1", "2" {
                    n449 = local write "Tab Control 2"(RANGE_Tab_Control_2."Meter 1 & 2" ("Tab Control 2")) -> ()
                  }
                }
              }
              frame True {
              }
            }
          }
        }
      }
      event "Meter 3/4": Value Change {
        n450 = event-data() -> ("NewVal"=w891:string)  [unwired: 1 in, 5 out]
        n451 = local read "Meter Select 2"() -> (w890:T5)
        n452 = case shown="\"Auto\"" w890 {
          tunnel: w891 -> [_ w898]
          frame Default {
          }
          frame "Auto" {
            n453 = local read "All Meter Data"() -> (w893:T13)
            n454 = Unbundle By Name(w893) -> ("Use Auto Switching"=w894:bool, "Meter Bank 2.Panel Data.Mass Flow"=w896:dbl)
            n455 = Greater Than 0?(x=w896) -> (x > 0?=w895:bool)
            n456 = And(x=w894, y=w895) -> (x .and. y?=w892:bool)
            n457 = case shown="True" w892 {
              tunnel: [TRUE w903] -> w897
              frame False {
              }
              frame True {
                n458 = local read "Tab Control 2"() -> (w901:T2)
                n459 = Equal?(x=w901, y=RANGE_Tab_Control_2."All Stations" ("Tab Control 2")) -> (x = y?=w905:bool)
                n460 = Equal?(x=w901, y=RANGE_Tab_Control_2."Custom Gases") -> (x = y?=w904:bool)
                n461 = Equal?(x=w901, y=RANGE_Tab_Control_2."Gas Valve Flow Test") -> (x = y?=w900:bool)
                n462 = Compound Arithmetic op=OR(w905, w904, w900) -> (w903:bool)
              }
            }
            n463 = case shown="False" w897 {
              tunnel: w898 -> [w908 _]
              frame False {
                n464 = case shown="\"3\", \"4\"" w908 {
                  frame Default {
                  }
                  frame "3", "4" {
                    n465 = local write "Tab Control 2"(RANGE_Tab_Control_2."Meter 3 & 4" ("Tab Control 2")) -> ()
                  }
                }
              }
              frame True {
              }
            }
          }
        }
      }
      event "Meter 5/6": Value Change {
        n466 = event-data() -> ("NewVal"=w911:string)  [unwired: 1 in, 5 out]
        n467 = local read "Meter Select 3"() -> (w910:T6)
        n468 = case shown="\"Auto\"" w910 {
          tunnel: w911 -> [_ w918]
          frame Default {
          }
          frame "Auto" {
            n469 = local read "All Meter Data"() -> (w913:T13)
            n470 = Unbundle By Name(w913) -> ("Use Auto Switching"=w914:bool, "Meter Bank 3.Panel Data.Mass Flow"=w916:dbl)
            n471 = Greater Than 0?(x=w916) -> (x > 0?=w915:bool)
            n472 = And(x=w914, y=w915) -> (x .and. y?=w912:bool)
            n473 = case shown="True" w912 {
              tunnel: [TRUE w923] -> w917
              frame False {
              }
              frame True {
                n474 = local read "Tab Control 2"() -> (w921:T2)
                n475 = Equal?(x=w921, y=RANGE_Tab_Control_2."All Stations" ("Tab Control 2")) -> (x = y?=w925:bool)
                n476 = Equal?(x=w921, y=RANGE_Tab_Control_2."Custom Gases") -> (x = y?=w924:bool)
                n477 = Equal?(x=w921, y=RANGE_Tab_Control_2."Gas Valve Flow Test") -> (x = y?=w920:bool)
                n478 = Compound Arithmetic op=OR(w925, w924, w920) -> (w923:bool)
              }
            }
            n479 = case shown="False" w917 {
              tunnel: w918 -> [w928 _]
              frame False {
                n480 = case shown="\"5\", \"6\"" w928 {
                  frame Default {
                  }
                  frame "5", "6" {
                    n481 = local write "Tab Control 2"(RANGE_Tab_Control_2."Meter 5 & 6" ("Tab Control 2")) -> ()
                  }
                }
              }
              frame True {
              }
            }
          }
        }
      }
    }
    n482 = call "UTILITY Boolean Notifier.vi"("Status"=UTILITY_Notifier."Read", "name (unnamed)"="Exit") -> ("latest READ notification"=w867:bool)  [unwired: 8 in, 1 out]
    "Event Loop" <- w866
  }
  n483 = while {
    tunnel: [w931] -> w13
    tunnel: w8 -> [w946]
    tunnel: w7 -> [w945]
    tunnel: w6 -> [w944]
    tunnel: [w943] -> w4
    tunnel: [w942] -> w5
    tunnel: w2 -> [w934]
    stop <- w939 stop-if-true
    # "HHV Loop"
    n484 = call "Inficon 32 Bit Data.vi"("HHV Manual Mode?"=w934, "Gas Type"=enum16{"Natural Gas", "Propane Gas"}."Natural Gas", "Error In"=w946, "Modbus master in"=w945) -> ("Error Out"=w949:errorcluster, "Inficon Data Output"=w938:T31, "Modbus master out"=w943:refnum<class "Modbus Master.lvclass">)  [unwired: 4 in, 1 out]
    n485 = Unbundle By Name(w938) -> ("Gross Heating Value, Vol (Real, Dry)"=→"HHV Natural Gas":dbl)
    n486 = call "Inficon 32 Bit Data.vi"("HHV Manual Mode?"=w934, "Gas Type"=enum16{"Natural Gas", "Propane Gas"}."Propane Gas", "Error In"=w949, "Modbus master in"=w944) -> ("Error Out"=w933:errorcluster, "Inficon Data Output"=w937:T31, "Modbus master out"=w942:refnum<class "Modbus Master.lvclass">)  [unwired: 4 in, 1 out]
    n487 = Unbundle By Name(w937) -> ("Gross Heating Value, Vol (Real, Dry)"=→"HHV Propane":dbl)
    n488 = call <vilib>:"Clear Errors.vi"("error in (no error)"=w933, "specific error code to clear (0: all)"=0) -> ("error out"=w931:errorcluster)  [unwired: 4 in, 1 out]
    n489 = call "UTILITY Boolean Notifier.vi"("Status"=UTILITY_Notifier."Read", "name (unnamed)"="Exit") -> ("latest READ notification"=w939:bool)  [unwired: 8 in, 1 out]
    n490 = Wait Until Next ms Multiple(millisecond multiple=u32 5000) -> ()  [unwired: 1 out]
  }
  n491 = while {
    tunnel: [w1035] -> w34
    shift-right: [w1047] -> _
    shift-left: w31 -> [w965]
    tunnel: w1 -> [w964]
    i -> [w1024]
    stop <- w1036 stop-if-true
    n492 = Bundle By Name(cluster=w965, "Threshold Voltage (NI DAQ)"="Rate Threshold (V)") -> (w1055:T13)
    n493 = local read "HHV Natural Gas"() -> (w955:dbl)
    n494 = local read "HHV Propane"() -> (w954:dbl)
    n495 = control-ref of="HeatingValueS3"() -> (w953:refnum<vi>)
    n496 = control-ref of="HeatingValueS2"() -> (w952:refnum<vi>)
    n497 = control-ref of="HeatingValueS1"() -> (w951:refnum<vi>)
    n498 = local read "Display Bank 3"() -> (w961:T7)
    n499 = local read "Display Bank 2"() -> (w962:T7)
    n500 = local read "Display Bank 1"() -> (w963:T7)
    n501 = call "RANGE Update HHV.vi"("HHV Propane"=w954, "HHV Ref"=w951, "HHV Natural Gas"=w955, "error in (no error)"=w964, "Manual HHV"="Manual HHV 1", "Display Bank"=w963) -> ("error out"=w960:errorcluster)  [unwired: 5 in]
    n502 = call "RANGE Update HHV.vi"("HHV Propane"=w954, "HHV Ref"=w952, "HHV Natural Gas"=w955, "error in (no error)"=w960, "Manual HHV"="Manual HHV 2", "Display Bank"=w962) -> ("error out"=w959:errorcluster)  [unwired: 5 in]
    n503 = call "RANGE Update HHV.vi"("HHV Propane"=w954, "HHV Ref"=w953, "HHV Natural Gas"=w955, "error in (no error)"=w959, "Manual HHV"="Manual HHV 3", "Display Bank"=w961) -> ("error out"=w950:errorcluster)  [unwired: 5 in]
    n504 = Bundle By Name(cluster=w1055, "Meter Bank 1.Panel Data.Heating Value (BTU/ft³)"="HeatingValueS1", "Meter Bank 2.Panel Data.Heating Value (BTU/ft³)"="HeatingValueS2", "Meter Bank 3.Panel Data.Heating Value (BTU/ft³)"="HeatingValueS3") -> (w1053:T13)
    n505 = local read "Tot.Flow (SLPM Liters) Bank 1"() -> (w1027:dbl)
    n506 = local read "Tot.Flow (SLPM Liters) Bank 2"() -> (w1026:dbl)
    n507 = local read "Tot.Flow (SLPM Liters) Bank 3"() -> (w1025:dbl)
    n508 = flat-sequence {
      tunnel: [w1062] -> w975
      tunnel: w950 -> [_]
      frame #0 {
        n509 = Get Date/Time In Seconds() -> (seconds since 1Jan1904=w1063:timestamp)
        n510 = To Double Precision Float(number=w1063) -> (double precision float=w1062:dbl)
      }
    }
    n511 = call "RANGE GET Gas Data.vi"("DAQ Data In"=w1053, "Tot.Flow (Liters) Bank 1"=w1027, "Tot.Flow (Liters) Bank 2"=w1026, "Tot.Flow (Liters) Bank 3"=w1025, "Error In"=w950, "Meter Select 3"="Meter Select 3", "Meter Select 2"="Meter Select 2", "Meter Select 1"="Meter Select") -> ("DAQ Data Out"=w1049:T13, "Error Out"=w978:errorcluster)  [unwired: 10 in]
    n512 = flat-sequence {
      tunnel: [w1060] -> w974
      tunnel: w978 -> [_]
      frame #0 {
        n513 = Get Date/Time In Seconds() -> (seconds since 1Jan1904=w1061:timestamp)
        n514 = To Double Precision Float(number=w1061) -> (double precision float=w1060:dbl)
      }
    }
    n515 = call "RANGE General Data Processing.vi"("DAQ Data Out in"=w1049, "Meter Select 3"="Meter Select 3", "Meter Select 2"="Meter Select 2", "Meter Select 1"="Meter Select", "error in (no error)"=w978) -> ("DAQ Data Out out"=w1046:T13, "error out"=w977:errorcluster)  [unwired: 9 in]
    n516 = local read "Average Updates"() -> (w1045:T13)
    n517 = flat-sequence {
      tunnel: [w1058] -> w973
      tunnel: w977 -> [_]
      frame #0 {
        n518 = Get Date/Time In Seconds() -> (seconds since 1Jan1904=w1059:timestamp)
        n519 = To Double Precision Float(number=w1059) -> (double precision float=w1058:dbl)
      }
    }
    n520 = local read "ANSI 3"() -> (w1031:bool)
    n521 = local read "ANSI 2"() -> (w1032:bool)
    n522 = local read "ANSI 1"() -> (w1033:bool)
    n523 = call "RANGE Update Averages.vi"("DAQ Data Out in"=w1046, "Average Updates"=w1045, "Error In"=w977, "Meter Bank 1.Start ANSI"=w1033, "Meter Bank 2.Start ANSI"=w1032, "Meter Bank 3.Start ANSI"=w1031) -> ("DAQ Data Out out"=w1047:T13, "Error Out"=w976:errorcluster)  [unwired: 12 in]
    "All Meter Data" <- w1047
    n524 = Unbundle By Name(w1047) -> ("Meter Bank 1.Flow Rate (BTU/HR)"=w1043:dbl, "Meter Bank 2.Flow Rate (BTU/HR)"=w1042:dbl, "Meter Bank 3.Flow Rate (BTU/HR)"=w1041:dbl, "Meter Bank 1.Panel Data"=→"Display Bank 1" →"Display S1":T7, "Meter Bank 2.Panel Data"=→"Display Bank 2" →"Display S2":T7, "Meter Bank 3.Panel Data"=→"Display Bank 3" →"Display S3":T7, "Meter Bank 1.Flow Rate (BTU/HR)"=w1052:dbl, "Meter Bank 2.Flow Rate (BTU/HR)"=w1051:dbl, "Meter Bank 3.Flow Rate (BTU/HR)"=w1050:dbl, "Meter Bank 1.Meter ID"=w1018:string, "Meter Bank 2.Meter ID"=w1007:string, "Meter Bank 3.Meter ID"=w1002:string, "Meter 1.Measurement Units"=w1020:T15, "Meter 2.Measurement Units"=w1019:T15, "Meter 3.Measurement Units"=w1006:T15, "Meter 4.Measurement Units"=w1005:T15, "Meter 5.Measurement Units"=w1004:T15, "Meter 6.Measurement Units"=w1003:T15)
    "Flow Rate S1" <- w1043
    "Flow Rate S2" <- w1042
    "Flow Rate S3" <- w1041
    n525 = flat-sequence {
      tunnel: [w1056] -> w972
      tunnel: w976 -> [_]
      frame #0 {
        n526 = Get Date/Time In Seconds() -> (seconds since 1Jan1904=w1057:timestamp)
        n527 = To Double Precision Float(number=w1057) -> (double precision float=w1056:dbl)
      }
    }
    n528 = while {
      tunnel: w1018 -> [w1143]
      shift-right: [w1142] -> _
      shift-left: _ -> [w1151]
      tunnel: w1007 -> [w1141]
      shift-right: [w1140] -> _
      shift-left: _ -> [w1150]
      tunnel: w1002 -> [w1144]
      shift-right: [w1139] -> _
      shift-left: _ -> [w1149]
      stop <- TRUE stop-if-true
      # "Auto Switch Tab FGV"
      n529 = Not Equal?(x=w1151, y=w1143) -> (x != y?=w1147:bool)
      n530 = Not Equal?(x=w1150, y=w1141) -> (x != y?=w1146:bool)
      n531 = Not Equal?(x=w1149, y=w1144) -> (x != y?=w1145:bool)
      n532 = Compound Arithmetic op=OR(w1147, w1146, w1145) -> (w1148:bool)
      n533 = case shown="True" w1148 {
        tunnel: w1143 -> [w1153 w1164]
        tunnel: w1147 -> [_ w1163]
        tunnel: w1146 -> [_ w1162]
        tunnel: w1141 -> [w1155 w1161]
        tunnel: w1145 -> [_ w1160]
        tunnel: w1144 -> [w1154 w1159]
        tunnel: [w1153 w1158] -> w1142
        tunnel: [w1155 w1157] -> w1140
        tunnel: [w1154 w1156] -> w1139
        frame False {
        }
        frame True {
          n534 = case shown="True" w1163 {
            tunnel: w1164 -> [w1179 w1182]
            tunnel: [w1179 "" ("Meter ID")] -> w1158
            frame False {
            }
            frame True {
              n535 = case shown="\"A\"" w1182 {
                selector: w1182 -> [w1183 _ _]
                tunnel: [w1183 "1" "2"] -> w1181
                frame Default {
                }
                frame "A" {
                }
                frame "B" {
                }
              }
              n536 = property on="Meter 1/2" class="Str"("Val(Sgnl)"=w1181) -> ()  [unwired: 2 in, 2 out]
            }
          }
          n537 = case shown="True" w1162 {
            tunnel: w1161 -> [w1172 w1175]
            tunnel: [w1172 "" ("Meter ID")] -> w1157
            frame False {
            }
            frame True {
              n538 = case shown="\"D\"" w1175 {
                selector: w1175 -> [w1176 _ _]
                tunnel: [w1176 "3" "4"] -> w1174
                frame Default {
                }
                frame "C" {
                }
                frame "D" {
                }
              }
              n539 = property on="Meter 3/4" class="Str"("Val(Sgnl)"=w1174) -> ()  [unwired: 2 in, 2 out]
            }
          }
          n540 = case shown="True" w1160 {
            tunnel: w1159 -> [w1165 w1168]
            tunnel: [w1165 "" ("Meter ID")] -> w1156
            frame False {
            }
            frame True {
              n541 = case shown="Default" w1168 {
                selector: w1168 -> [w1169 _ _]
                tunnel: [w1169 "5" "6"] -> w1167
                frame Default {
                }
                frame "E" {
                }
                frame "F" {
                }
              }
              n542 = property on="Meter 5/6" class="Str"("Val(Sgnl)"=w1167) -> ()  [unwired: 2 in, 2 out]
            }
          }
        }
      }
    }
    n543 = call <vilib>:"Clear Errors.vi"("error in (no error)"=w976) -> ("error out"=w1034:errorcluster)  [unwired: 5 in, 1 out]
    n544 = Subtract(x=w974, y=w975) -> (x-y=→"Get Gas Data Time":dbl)
    n545 = Subtract(x=w973, y=w974) -> (x-y=→"Data Process Time":dbl)
    n546 = local write "Flow Rate"(w1043) -> ()
    n547 = Bundle("Flow Rate (BTU/HR)"=w1052) -> (→"DisplayChart" →"Station 1 Chart":cluster{"Flow Rate (BTU/HR)":dbl})  [unwired: 1 in]
    n548 = Bundle("Flow Rate (BTU/HR)"=w1051) -> (→"DisplayChart 2" →"Station 2 Chart":cluster{"Flow Rate (BTU/HR)":dbl})  [unwired: 1 in]
    n549 = Bundle("Flow Rate (BTU/HR)"=w1050) -> (→"DisplayChart 3" →"Station 3 Chart":cluster{"Flow Rate (BTU/HR)":dbl})  [unwired: 1 in]
    n550 = case shown="\"C\"" w1007 {
      tunnel: w1006 -> [w1090 _ _]
      tunnel: w1005 -> [_ w1102 _]
      tunnel: [w1100 w1112 w1113] -> w1001
      tunnel: [w1099 w1111 w1113] -> w1000
      tunnel: [w1098 w1110 w1113] -> w999
      tunnel: [w1097 w1109 w1113] -> w998
      tunnel: [w1096 w1108 w1113] -> w997
      tunnel: [w1095 w1107 w1113] -> w996
      tunnel: [w1094 w1106 w1113] -> w995
      tunnel: [w1093 w1105 w1113] -> w994
      tunnel: [w1092 w1104 w1113] -> w993
      tunnel: [w1091 w1103 w1113] -> w992
      tunnel: [w1089 w1101 w1113] -> w980
      frame "C" {
        n551 = Unbundle By Name(w1090) -> ("Units of Measure Input.Abs. Pressure"=w1100:string, "Units of Measure Input.Temperature"=w1099:string, "Units of Measure Input.Volume"=w1098:string, "Units of Measure Input.Mass"=w1097:string, "Units of Measure Input.Totalizer"=w1096:string)
        n552 = Unbundle By Name(w1090) -> ("Units of Measure Input.Abs. Pressure"=w1095:string, "Units of Measure Input.Temperature"=w1094:string, "Units of Measure Input.Volume"=w1093:string, "Units of Measure Input.Mass"=w1092:string, "Units of Measure Input.Totalizer"=w1091:string, "Software Rev"=w1089:string)
      }
      frame "D" {
        n553 = Unbundle By Name(w1102) -> ("Units of Measure Input.Abs. Pressure"=w1112:string, "Units of Measure Input.Temperature"=w1111:string, "Units of Measure Input.Volume"=w1110:string, "Units of Measure Input.Mass"=w1109:string, "Units of Measure Input.Totalizer"=w1108:string)
        n554 = Unbundle By Name(w1102) -> ("Units of Measure Input.Abs. Pressure"=w1107:string, "Units of Measure Input.Temperature"=w1106:string, "Units of Measure Input.Volume"=w1105:string, "Units of Measure Input.Mass"=w1104:string, "Units of Measure Input.Totalizer"=w1103:string, "Software Rev"=w1101:string)
      }
      frame Default {
        w1113 = "" ("Abs. Pressure")
      }
    }
    "Bank 2 Mass Flow" <- w998
    "Bank 2 Vol Flow" <- w999
    "Bank 2 Tot. Flow" <- w997
    "Bank 2 Gas Temp" <- w1000
    "Bank 2 Gas Pres" <- w1001
    "Bank 2 Mass Flow 2" <- w993
    "Bank 2 Vol Flow 3" <- w994
    "Bank 2 Tot. Flow 3" <- w992
    "Bank 2 Gas Temp 3" <- w995
    "Bank 2 Gas Pres 3" <- w996
    "Meter Software 3/4" <- w980
    n555 = case shown="\"E\"" w1002 {
      tunnel: w1004 -> [w1065 _ _]
      tunnel: w1003 -> [_ w1077 _]
      tunnel: [w1075 w1087 w1088] -> w991
      tunnel: [w1074 w1086 w1088] -> w990
      tunnel: [w1073 w1085 w1088] -> w989
      tunnel: [w1072 w1084 w1088] -> w988
      tunnel: [w1071 w1083 w1088] -> w987
      tunnel: [w1070 w1082 w1088] -> w986
      tunnel: [w1069 w1081 w1088] -> w985
      tunnel: [w1068 w1080 w1088] -> w984
      tunnel: [w1067 w1079 w1088] -> w983
      tunnel: [w1066 w1078 w1088] -> w982
      tunnel: [w1064 w1076 w1088] -> w979
      frame "E" {
        n556 = Unbundle By Name(w1065) -> ("Units of Measure Input.Abs. Pressure"=w1075:string, "Units of Measure Input.Temperature"=w1074:string, "Units of Measure Input.Volume"=w1073:string, "Units of Measure Input.Mass"=w1072:string, "Units of Measure Input.Totalizer"=w1071:string)
        n557 = Unbundle By Name(w1065) -> ("Units of Measure Input.Abs. Pressure"=w1070:string, "Units of Measure Input.Temperature"=w1069:string, "Units of Measure Input.Volume"=w1068:string, "Units of Measure Input.Mass"=w1067:string, "Units of Measure Input.Totalizer"=w1066:string, "Software Rev"=w1064:string)
      }
      frame "F" {
        n558 = Unbundle By Name(w1077) -> ("Units of Measure Input.Abs. Pressure"=w1087:string, "Units of Measure Input.Temperature"=w1086:string, "Units of Measure Input.Volume"=w1085:string, "Units of Measure Input.Mass"=w1084:string, "Units of Measure Input.Totalizer"=w1083:string)
        n559 = Unbundle By Name(w1077) -> ("Units of Measure Input.Abs. Pressure"=w1082:string, "Units of Measure Input.Temperature"=w1081:string, "Units of Measure Input.Volume"=w1080:string, "Units of Measure Input.Mass"=w1079:string, "Units of Measure Input.Totalizer"=w1078:string, "Software Rev"=w1076:string)
      }
      frame Default {
        w1088 = "" ("Abs. Pressure")
      }
    }
    "Bank 3 Mass Flow 2" <- w988
    "Bank 3 Vol Flow 2" <- w989
    "Bank 3 Tot. Flow 2" <- w987
    "Bank 3 Gas Temp 2" <- w990
    "Bank 3 Gas Pres 2" <- w991
    "Bank 3 Mass Flow" <- w983
    "Bank 3 Vol Flow" <- w984
    "Bank 3 Gas Temp" <- w985
    "Bank 3 Gas Pres" <- w986
    "Bank 3 Tot. Flow" <- w982
    "Meter Software 5/6" <- w979
    n560 = case shown="\"B\"" w1018 {
      tunnel: w1020 -> [w1115 _ _]
      tunnel: w1019 -> [_ w1127 _]
      tunnel: [w1125 w1137 w1138] -> w1017
      tunnel: [w1124 w1136 w1138] -> w1016
      tunnel: [w1123 w1135 w1138] -> w1015
      tunnel: [w1122 w1134 w1138] -> w1014
      tunnel: [w1121 w1133 w1138] -> w1013
      tunnel: [w1120 w1132 w1138] -> w1012
      tunnel: [w1119 w1131 w1138] -> w1011
      tunnel: [w1118 w1130 w1138] -> w1010
      tunnel: [w1117 w1129 w1138] -> w1009
      tunnel: [w1116 w1128 w1138] -> w1008
      tunnel: [w1114 w1126 w1138] -> w981
      frame "A" {
        n561 = Unbundle By Name(w1115) -> ("Units of Measure Input.Abs. Pressure"=w1125:string, "Units of Measure Input.Temperature"=w1124:string, "Units of Measure Input.Volume"=w1123:string, "Units of Measure Input.Mass"=w1122:string, "Units of Measure Input.Totalizer"=w1121:string)
        n562 = Unbundle By Name(w1115) -> ("Units of Measure Input.Abs. Pressure"=w1120:string, "Units of Measure Input.Temperature"=w1119:string, "Units of Measure Input.Volume"=w1118:string, "Units of Measure Input.Mass"=w1117:string, "Units of Measure Input.Totalizer"=w1116:string, "Software Rev"=w1114:string)
      }
      frame "B" {
        n563 = Unbundle By Name(w1127) -> ("Units of Measure Input.Abs. Pressure"=w1137:string, "Units of Measure Input.Temperature"=w1136:string, "Units of Measure Input.Volume"=w1135:string, "Units of Measure Input.Mass"=w1134:string, "Units of Measure Input.Totalizer"=w1133:string)
        n564 = Unbundle By Name(w1127) -> ("Units of Measure Input.Abs. Pressure"=w1132:string, "Units of Measure Input.Temperature"=w1131:string, "Units of Measure Input.Volume"=w1130:string, "Units of Measure Input.Mass"=w1129:string, "Units of Measure Input.Totalizer"=w1128:string, "Software Rev"=w1126:string)
      }
      frame Default {
        w1138 = "" ("Abs. Pressure")
      }
    }
    "Bank 1 Mass Flow 2" <- w1014
    "Bank 1 Vol Flow 2" <- w1015
    "Bank 1 Tot. Flow 2" <- w1013
    "Bank 1 Gas Temp 2" <- w1016
    "Bank 1 Gas Pres 2" <- w1017
    "Bank 1 Mass Flow" <- w1009
    "Bank 1 Vol Flow" <- w1010
    "Bank 1 Gas Temp" <- w1011
    "Bank 1 Gas Pres" <- w1012
    "Bank 1 Tot. Flow" <- w1008
    "Meter Software 1/2" <- w981
    n565 = Subtract(x=w972, y=w973) -> (x-y=→"Update Avg Time":dbl)
    n566 = local write "Flow Rate 2"(w1042) -> ()
    n567 = call "UTILITY Boolean Notifier.vi"("Status"=UTILITY_Notifier."Read", "error in (no error)"=w1034, "name (unnamed)"="Exit") -> ("error out"=w1035:errorcluster, "latest READ notification"=w1036:bool)  [unwired: 7 in]
    n568 = local write "Flow Rate 3"(w1041) -> ()
    n569 = Wait (ms)(milliseconds to wait=u32 250 ("millisecond multiple")) -> ()  [unwired: 1 out]
    "Main Control Loop" <- w1024
  }
  n570 = while {
    tunnel: w1 -> [w1186]
    tunnel: [w1186] -> w23
    i -> [w1187]
    stop <- w1194 stop-if-true
    n571 = local read "File Path"() -> (w1188:path)
    n572 = Equal?(x=w1188, y=path "") -> (x = y?=w1189:bool)
    n573 = case shown="False" w1189 {
      tunnel: w1188 -> [w1197 _]
      frame False {
        n574 = local read "All Meter Data"() -> (w1199:T13)
        n575 = local read "Elapsed Time"() -> (w1198:dbl)
        n576 = call "RANGE Write To File.vi"("Time"=w1198, "All Meter Data"=w1199, "File Path"=w1197) -> ()  [unwired: 8 in, 1 out]
      }
      frame True {
      }
    }
    n577 = call "UTILITY Boolean Notifier.vi"("Status"=UTILITY_Notifier."Read", "name (unnamed)"="Exit") -> ("latest READ notification"=w1194:bool)  [unwired: 8 in, 1 out]
    n578 = Multiply(x=T32 1000.0 ("y"), y="Scan Rate (Sec)") -> (x*y=w1191:T32)
    n579 = Wait (ms)(milliseconds to wait=w1191) -> ()  [unwired: 1 out]
    "Save Loop" <- w1187
  }
  n580 = while {
    shift-right: [w1214] -> _
    shift-left: w32 -> [w1217]
    shift-right: [w1213] -> _
    shift-left: w32 -> [w1216]
    shift-right: [w1212] -> _
    shift-left: w32 -> [w1215]
    tunnel: w1 -> [w1219]
    tunnel: [w1200] -> w25
    i -> [w1202]
    stop <- w1203 stop-if-true
    # "Integrate SLPM becasue it accounts for STP"
    n581 = local read "All Meter Data"() -> (w1220:T13)
    n582 = Unbundle By Name(w1220) -> ("Meter Bank 1.Panel Data.Mass Flow"=w1208:dbl, "Meter Bank 2.Panel Data.Mass Flow"=w1207:dbl, "Meter Bank 3.Panel Data.Mass Flow"=w1206:dbl)
    n583 = call "FMA1600A Get Bank Total Flow.vi"("Integral Array Input 1"=w1217, "Integral Array Input 2"=w1216, "Integral Array Input -3"=w1215, "Min to Sec Convert (Total Flow)"="Min to Sec Convert (Total Flow)", "error in (no error)"=w1219, "LPM (Vol. Flow) 1"=w1208, "LPM (Vol. Flow) 2"=w1207, "LPM (Vol. Flow) 3"=w1206) -> ("Tot.Flow (Liters) Bank 1"=→"Tot.Flow (SLPM Liters) Bank 1":dbl, "Tot.Flow (Liters) Bank 2"=→"Tot.Flow (SLPM Liters) Bank 2":dbl, "Tot.Flow (Liters) Bank 3"=→"Tot.Flow (SLPM Liters) Bank 3":dbl, "Integral Array Output 1"=w1214:dbl[], "Integral Array Output 2"=w1213:dbl[], "Integral Array Output-3"=w1212:dbl[], "error out"=w1201:errorcluster)  [unwired: 1 in]
    n584 = call "UTILITY Boolean Notifier.vi"("Status"=UTILITY_Notifier."Read", "error in (no error)"=w1201, "name (unnamed)"="Exit") -> ("error out"=w1200:errorcluster, "latest READ notification"=w1203:bool)  [unwired: 7 in]
    "Gas Total Loop" <- w1202
  }
  n585 = call-dynamic "Shutdown.vi"("error in"=w13, "Modbus master in"=w5) -> ("error out"=w15:errorcluster)  [unwired: 9 in]
  n586 = call-dynamic "Shutdown.vi"("error in"=w15, "Modbus master in"=w4) -> ("error out"=w3:errorcluster)  [unwired: 9 in]
  n587 = Merge Errors(w16, w23, w22, w25, w33, w34, w3) -> (w26:errorcluster)
  n588 = call <vilib>:"Clear Errors.vi"("error in (no error)"=w26) -> ("error out"=w14:errorcluster)  [unwired: 5 in, 1 out]
  n589 = call "UTILITY Boolean Notifier.vi"("Status"=UTILITY_Notifier."Release Ref", "error in (no error)"=w14, "Set Status"=FALSE, "name (unnamed)"="Exit") -> ("error out"=→"Error Out":errorcluster)  [unwired: 6 in, 1 out]
